vi "Steuerprogramm-12-15.vi"() -> ()   [LabVIEW 2010]
uses:
  <vilib>/rvi/interface/nirviReadWriteControl/nirviReadWriteControl.xnode
  <vilib>/rvi/errors/niLvFpgaWhatHappensToTopLevelVI.ctl
  <vilib>/rvi/interface/common/niFpgaNodeNameForErrorReporting.ctl
  <vilib>/rvi/errors/niLvFpgaAdjustHostInterfaceError.vi
  gvbooleschRT.vi
  <vilib>/rvi/interface/nirviCloseFPGA/nirviCloseFPGA.xnode
  GVMWHorst.vi
  GVMethodenwechsel.vi
  GVHorstSP.vi
  GVZwangs.vi
  GVHK1Hz.vi
  GVHeizenLH.vi
  GVAIs.vi
  GVTrapsMachs.vi
  GVaktuelleTDMS.vi
  GVECDs.vi
  GVZeitenZyklen.vi
  GVProbenvol.vi
  GVVentilposition.vi
  <vilib>/rvi/interface/nirviMethod/nirviMethod.xnode
  GVChroms.vi
  C:/Users/HAGAR-IV/Desktop/Zeugs/Johnny/pertrasgc fpga/FPGA-Programm-11-15.vi
  GVMetavariablen.vi
  GVZwangsMPV.vi
  C:/Users/HAGAR-IV/Desktop/Zeugs/markus/version feb 2012/FPGA Bitfiles/pertrasgcfpga2_FPGATarget_FPGA-Programm-11_875D3646.lvbitx
  NiFpgaLv.dll
  <vilib>/Utility/error.llb/Error Cluster From Error Code.vi
  <vilib>/FPGAPlugInAG/cRIO-9114/niLvFpga_Close_cRIO-9114.vi
  Emil/HAGAR V - Licor/control/Licor-Sequences.ctl
  Emil/HAGAR V - Licor/control/Licor-Pump.ctl
  Emil/Licor-Steuerung/LicorLI7000/conventions/Licor-Source.ctl
  Emil/Licor-Steuerung/LicorLI7000/LicorLI7000.lvlib
  Emil/HAGAR V - Licor/control/Licor-Parameter.ctl
panel:
  in  "Methode speichern":bool
  out "ZyklusNummernGesamt":i32[](array[numeric])
  in  "veränderte Methode benutzen":bool
  in  "Methode verändern":bool
  out "ZyklusNummern":i32[](array[numeric])
  out "Big Ben, Methodenzeit, Zykluszeit0, Zykluszeit1, Zykluszeit2A, Zykluszeit2B":i32[](array[numeric])
  in  "global stop RT":bool
  in  "Methode":i32(ring) items=["Bedingsmethode", "Startmethode", "Meßmodus", "Shut-up-Methode", "Test", "HAG2 1/2", "Startmethode", "HAG2 1/2 Aufwärmen"]
  in  "Registerkarte":T1(tab)
  out "AIs1":dbl[](array[numeric])
  out "AIs1":string[](array[string])
  out "AIs2":string[](array[string])
  out "AIs3":string[](array[string])
  out "AIs2":dbl[](array[numeric])
  out "AIs3":dbl[](array[numeric])
  out "Metavariablen":string[](array[string])
  out "Metavariablen":dbl[](array[numeric])
  out "MWHorst":dbl[](array[numeric])
  out "HorstRegler":string[](array[string])
  out "Ventilposition":i32=1 min=1 max=6 step=1
  out "Housekeeping1":cluster{dbl[], dbl[]}(graph)
  in  "Zeitachse1":i32(ring)=1 items=["Zykluszeit [s] Mod0", "Zykluszeit [s] Mod1", "Zykluszeit [s] Mod2A", "Zykluszeit [s] Mod2B"]
  in  "dargestellte Größe 1":i32(ring)=1 items=["T1-Trap1", "T1-Trap2", "T1-StirlingKühlkopf", "T1-PreCol1", "T1-PreCol2", "T1-MainCol1a", "T1-MainCol1b", "T1-MainCol2a", "T1-MainCol2b", "T1-Bronkhorst1a", "T1-Bronkhorst1b", "T1-Bronkhorst2a", "T1-Bronkhorst2b", "T1-2Pos1B", "T1-Spare9", "T1-2Pos1A", "T1-Spare10", "T1-TurboPump", "T1-StirlingPlatine", "T1-Spare5", "T1-Spare6", "T1-Spare7", "T1-Spare8", "F1-MFM1", "F1-MFM0D [mL]", "P1-MethaneHP", "P1-MethaneLP", "P1-Vacuum", "TurboSpeed", "I1-MS-AC", "I1-Trap1", "I1-Trap2", "T2-ECD1a", "T2-ECD1b", "T2-ECD2a", "T2-ECD2b", "T2-Col1a", "T2-Col1b", "T2-Col2a", "T2-Col2b", "T2-Spare1", "T2-Spare2", "T2-Oven_a", "T2-Oven_b", "T2-Spare3", "T2-Spare4", "T2-Spare5", "F2-MFM0", "F2-MFM2A", "F2-MFM2B", "P2-N2O_HP", "P2-N2O_LP", "P2-CO2_HP", "P2-CO2_LP", "AI-Spare1", "FL-MFM1000mL", "AI-Spare3", "AI-Spare4", "StirlingAlarm", "StirlingEmerg.", "AI-Spare7", "AI-Spare8", "AI-Spare9", "FL-MFM30mL", "T0-DC/DC5", "I0-24V_M0", "I0-48V_M1", "I0-24V_M1", "I0-28V_M2", "T0-Spare3", "T0-Spare2", "T0-Spare4", "T0-DC/DC7", "I0-20V_Laptop", "I0-28V_M1", "I0-24V_M2", "I0-12V_Licor", "T0-Spare1", "T0-Drier", "T0-Spare5", "F0-MFM0A [L]", "TL-Licor_a", "P0-Span-HP", "P0-spare1", "P0-Stickstoff-LP", "P0-Helium-LP", "P0-Cal-HP", "P0-P9Tavco[bar]", "F0-MFM0B [L]", "TL-Licor_b", "P0-Span-LP", "P0-spare2", "P0-Stickstoff-HP", "P0-Helium-HP", "P0-Cal-LP", "F0-MFM3", "TemperaturTrap1[°C]", "TemperaturTrap2[°C]", "TemperaturPreMach1[°C]", "TemperaturPreMach2[°C]", "TemperaturMainMach1[°C]", "TemperaturMainMach2[°C]", "PrC0", "PrC0-Licor", "PrC1-Säule2", "PrC1-Säule1", "MFC1-Sample", "MFC1-Methan", "PrC1-BackFlush1", "PrC1-BackFlush2", "MFC2A", "MFC2B", "MFC2C", "PrC2A", "MFC2D", "MFC2E", "PrC2B"]
  out "Housekeeping2":cluster{dbl[], dbl[]}(graph)
  in  "Zeitachse2":i32(ring)=1 items=["Zykluszeit [s] Mod0", "Zykluszeit [s] Mod1", "Zykluszeit [s] Mod2A", "Zykluszeit [s] Mod2B"]
  in  "dargestellte Größe 2":i32(ring)=1 items=["T1-Trap1", "T1-Trap2", "T1-StirlingKühlkopf", "T1-PreCol1", "T1-PreCol2", "T1-MainCol1a", "T1-MainCol1b", "T1-MainCol2a", "T1-MainCol2b", "T1-Bronkhorst1a", "T1-Bronkhorst1b", "T1-Bronkhorst2a", "T1-Bronkhorst2b", "T1-2Pos1B", "T1-Spare9", "T1-2Pos1A", "T1-Spare10", "T1-TurboPump", "T1-StirlingPlatine", "T1-Spare5", "T1-Spare6", "T1-Spare7", "T1-Spare8", "F1-MFM1", "F1-MFM0D [mL]", "P1-MethaneHP", "P1-MethaneLP", "P1-Vacuum", "TurboSpeed", "I1-MS-AC", "I1-Trap1", "I1-Trap2", "T2-ECD1a", "T2-ECD1b", "T2-ECD2a", "T2-ECD2b", "T2-Col1a", "T2-Col1b", "T2-Col2a", "T2-Col2b", "T2-Spare1", "T2-Spare2", "T2-Oven_a", "T2-Oven_b", "T2-Spare3", "T2-Spare4", "T2-Spare5", "F2-MFM0", "F2-MFM2A", "F2-MFM2B", "P2-N2O_HP", "P2-N2O_LP", "P2-CO2_HP", "P2-CO2_LP", "AI-Spare1", "FL-MFM1000mL", "AI-Spare3", "AI-Spare4", "StirlingAlarm", "StirlingEmerg.", "AI-Spare7", "AI-Spare8", "AI-Spare9", "FL-MFM30mL", "T0-DC/DC5", "I0-24V_M0", "I0-48V_M1", "I0-24V_M1", "I0-28V_M2", "T0-Spare3", "T0-Spare2", "T0-Spare4", "T0-DC/DC7", "I0-20V_Laptop", "I0-28V_M1", "I0-24V_M2", "I0-12V_Licor", "T0-Spare1", "T0-Drier", "T0-Spare5", "F0-MFM0A [L]", "TL-Licor_a", "P0-Span-HP", "P0-spare1", "P0-Stickstoff-LP", "P0-Helium-LP", "P0-Cal-HP", "P0-P9Tavco[bar]", "F0-MFM0B [L]", "TL-Licor_b", "P0-Span-LP", "P0-spare2", "P0-Stickstoff-HP", "P0-Helium-HP", "P0-Cal-LP", "F0-MFM3", "TemperaturTrap1[°C]", "TemperaturTrap2[°C]", "TemperaturPreMach1[°C]", "TemperaturPreMach2[°C]", "TemperaturMainMach1[°C]", "TemperaturMainMach2[°C]", "PrC0", "PrC0-Licor", "PrC1-Säule2", "PrC1-Säule1", "MFC1-Sample", "MFC1-Methan", "PrC1-BackFlush1", "PrC1-BackFlush2", "MFC2A", "MFC2B", "MFC2C", "PrC2A", "MFC2D", "MFC2E", "PrC2B"]
  out "Detektor 2":cluster{dbl[], dbl[]}[](graph)
  in  "Detektor":i32(ring) items=["ECD1", "ECD2"]
  in  "HK1YMin":dbl
  in  "HK1YMax":dbl=100.0
  in  "HK2YMin":dbl
  in  "HK2YMax":dbl=100.0
  in  "DetYMin":dbl
  in  "DetYMax":dbl=100.0
  out "schnelleAnzeige":cluster{dbl[], dbl[]}(graph)
  in  "TafelWischen!":bool
  in  "dargestellte Größe 3":i32(ring)=1 items=["TemperaturTrap1[°C]", "TemperaturTrap2[°C]", "TemperaturPreMach1[°C]", "TemperaturPreMach2[°C]", "TemperaturMainMach1[°C]", "TemperaturMainMach2[°C]", "PrC0", "PrC0-Licor", "PrC1-Säule2", "PrC1-Säule1", "MFC1-Sample", "MFC1-Methan", "PrC1-BackFlush1", "PrC1-BackFlush2", "MFC2A", "MFC2B", "MFC2C", "PrC2A", "MFC2D", "MFC2E", "PrC2B"]
  in  "An/Aus":bool
  in  "manual control":T3={"sequence manual"=enum."WAIT", "sequence manual ?"=FALSE}
  out "Licor-output":string[](array[string])
  out "graph":cluster{"X":dbl[], "Y":dbl[]}(graph)
  in  "Licor-parameter out":T4={"CO2 ref"=392.0, "CO2 span"=402.0, "H2O ref"=0.0, "H2O span"=0.0, "Zi"=1.2, "Zt"=0.0, "Zm"=0.0, "S"=1.0, "Temp [C]"=50.0, "Pressure [hPa]"=135.0, "Licor-Sources"=["CO2A W", "CO2B W", "H2OA W", "H2OB W", "T C", "T V", "P kPa", "P V", "RH %", "CO2A um/m", "CO2B um/m", "H2OA mm/m", "H2OB mm/m"], "Licor-Pump"="Off", "Zeitstempel"=timestamp(0 s since 1904-01-01)} {"Pressure [hPa]" format="%.2g"; "Temp [C]" format="%.2f"; "CO2 ref" format="%.2f"; "CO2 span" format="%.2g"; "H2O ref" format="%.2g"; "H2O span" format="%.2g"}
  in  "ServosWarmHigh (us)KaltHigh(us)":T7={"Servo1WarmHigh(us)"=1000, "Servo1KaltHigh(us)"=1000, "Servo2WarmHigh(us)"=2030, "Servo2KaltHigh(us)"=2030}
  out "KonfigLaden":errorcluster
  out "FPGAInit":errorcluster
  out "TDMSwriteECD1":errorcluster
  out "TDMSwriteECD2":errorcluster
  out "AIsFIFOread":errorcluster
  out "MWTrapsMachs":errorcluster
  out "TDMSwriteHK":errorcluster
  out "TDMSopenHK":errorcluster
  out "TDMScloseHK":errorcluster
  out "writeFIFORS485":errorcluster
  out "SeriellReadWrite":errorcluster
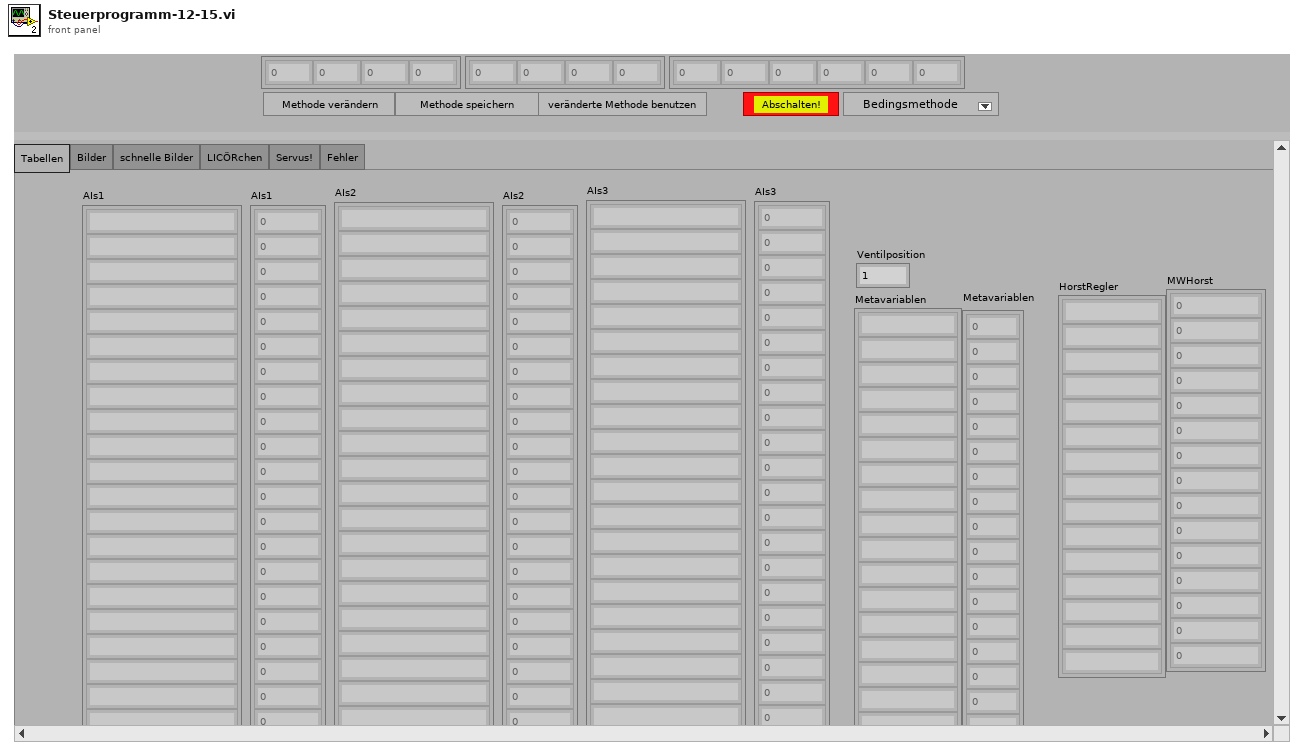
[diagram p1: front panel]
types:
  T1 = enum32{"Tabellen", "Bilder", "schnelle Bilder", "LICÖRchen", "Servus!", "Fehler"}
  T2 = typedef "Licor-Sequences.ctl" = enum16{"test", "WAIT", "warmup", "initialize", "calibrate Z", "calibrate S"}
  T3 = cluster{"sequence manual":T2, "sequence manual ?":bool}
  T4 = typedef "Licor-Parameter.ctl" = cluster{"CO2 ref":dbl, "CO2 span":dbl, "H2O ref":dbl, "H2O span":dbl, "Zi":dbl, "Zt":dbl, "Zm":dbl, "S":dbl, "Temp [C]":dbl, "Pressure [hPa]":dbl, "Licor-Sources":T5[], "Licor-Pump":T6, "Zeitstempel":timestamp}
  T5 = typedef "LicorLI7000.lvlib/Licor-Source.ctl" = string
  T6 = typedef "Licor-Pump.ctl" = string
  T7 = cluster{"Servo1WarmHigh(us)":u32, "Servo1KaltHigh(us)":u32, "Servo2WarmHigh(us)":u32, "Servo2KaltHigh(us)":u32}
  T8 = cluster{"DIOsMod0Nr":i32[], "DIOsMod1Nr":i32[], "DIOsMod2ANr":i32[], "DIOsMod2BNr":i32[], "AIsLH":i32[], "AnzahlRegler/Modul":i32[], "Regler für den Probenfluß":i32, "SPvorgebenMod0":string[], "SPvorgebenMod1":string[], "SPvorgebenMod2A":string[], "SPvorgebenMod2B":string[], "MWAntwortMod0":string[], "MWAntwortMod1":string[], "MWAntwortMod2A":string[], "MWAntwortMod2B":string[], "FaktorMod0":dbl[], "FaktorMod1":dbl[], "FaktorMod2A":dbl[], "FaktorMod2B":dbl[], "MWabfragenMod0":string[], "MWabfragenMod1":string[], "MWabfragenMod2A":string[], "MWabfragenMod2B":string[], "Modul1/AI koeff":dbl[][], "Modul2/AI koeff":dbl[][], "Modul3/AI koeff":dbl[][], "Traps/MachsKoeff":dbl[][], "Modul1/AIsNamen":string[], "Modul2/AIsNamen":string[], "Modul3/AIsNamen":string[], "DIOsMod0Name":string[], "DIOsMod1Name":string[], "DIOsMod2AName":string[], "DIOsMod2BName":string[], "ReglerNameMod0":string[], "ReglerNameMod1":string[], "ReglerNameMod2A":string[], "ReglerNameMod2B":string[], "Startmethode":i32, "Dateiordner Housekeeping":path, "Dateiname Housekeeping":string, "DateiordnerECD1":path, "DateinameECD1":string, "DateiordnerECD2":path, "DateinameECD2":string, "NamenLangsameHeizungen":string[], "ModuleLH":i32[], "Metavariablen":string[]}
  T9 = cluster{"Zykluslängen [s]":dbl[], "ZeitpktDIOsMod0":dbl[], "ZeitpktDIOsMod1":dbl[], "ZeitpktDIOsMod2A":dbl[], "ZeitpktDIOsMod2B":dbl[], "DIOsSPMod0":bool[][], "DIOsSPMod1":bool[][], "DIOsSPMod2A":bool[][], "DIOsSPMod2B":bool[][], "Mod0HorstZeitpkt":dbl[], "Mod1HorstZeitpkt":dbl[], "Mod2AHorstZeitpkt":dbl[], "Mod2BHorstZeitpkt":dbl[], "HorstSPMod0":dbl[][], "HorstSPMod1":dbl[][], "HorstSPMod2A":dbl[][], "HorstSPMod2B":dbl[][], "LHSetpoints":dbl[], "LHHeizen?":bool[], "ZPktFPGABoolesch":dbl[], "FPGABoolesch":bool[][], "ZeitpktFPGAPID":dbl[], "FPGAPID":cluster{"proportional gain (Kc)":fxp<+/-,16,8>, "integral gain (Kc*Ts/Ti)":fxp<+/-,16,8>, "derivative gain (Kc*Td/Ts)":fxp<+/-,16,8>}[][], "ZeitpktFPGAFixp":dbl[], "SHSetpoints":dbl[][], "t_PreMach1":dbl[], "T_PreMach1":dbl[], "t_PreMach2":dbl[], "T_PreMach2":dbl[], "PIDs für \"träge\" Heizungen":cluster{"proportional gain (Kc)":dbl, "integral time (Ti, min)":dbl, "derivative time (Td, min)":dbl}[], "Zwangsbedingungen":dbl[][], "Dateien fürs MS schicken?":bool, "ZeitpunkteMPV":dbl[], "SPMPV":i32[], "ZeitpktMS-1":dbl, "ZeitpktMS-2":dbl, "Int.Start1":dbl, "Int.Stop1":dbl, "Int.Start2":dbl, "Int.Stop2":dbl, "Methodenname":string, "t_MainMach1":dbl[], "T_MainMach1":dbl[], "t_MainMach2":dbl[], "T_MainMach2":dbl[]}[]
  T10 = enum16{"open", "replace", "create", "open or create", "replace or create", "replace or create with confirmation"}
  T11 = typedef "niFpgaNodeNameForErrorReporting.ctl" = enum16{"Open FPGA VI Reference", "Read/Write Control", "Invoke Method: Abort", "Invoke Method: Acknowledge IRQ", "Invoke Method: Download", "Invoke Method: FIFO.Configure", "Invoke Method: FIFO.Read", "Invoke Method: FIFO.Start", "Invoke Method: FIFO.Stop", "Invoke Method: FIFO.Write", "Invoke Method: Reset", "Invoke Method: Run", "Invoke Method: Wait on IRQ", "Close FPGA VI Reference"}
  T12 = typedef "niLvFpgaWhatHappensToTopLevelVI.ctl" = enum16{"top level VI scripted behind XNode", "top level VI inlined behind XNode"}
  T13 = cluster{"Zyklus1":i32, "Zeitachse1":i32, "dargestellte Größe 1":i32, "Zyklus2":i32, "Zeitachse2":i32, "dargestellte Größe 2":i32}
  T14 = cluster{"DIOsMod0Name":string[], "DIOsMod1Name":string[], "DIOsMod2AName":string[], "DIOsMod2BName":string[], "ReglerNameMod0":string[], "ReglerNameMod1":string[], "ReglerNameMod2A":string[], "ReglerNameMod2B":string[], "NamenLangsameHeizungen":string[]}
  T15 = cluster{"Zykluslängen [s]":dbl[], "ZeitpktDIOsMod0":dbl[], "ZeitpktDIOsMod1":dbl[], "ZeitpktDIOsMod2A":dbl[], "ZeitpktDIOsMod2B":dbl[], "DIOsSPMod0":bool[][], "DIOsSPMod1":bool[][], "DIOsSPMod2A":bool[][], "DIOsSPMod2B":bool[][], "Mod0HorstZeitpkt":dbl[], "Mod1HorstZeitpkt":dbl[], "Mod2AHorstZeitpkt":dbl[], "Mod2BHorstZeitpkt":dbl[], "HorstSPMod0":dbl[][], "HorstSPMod1":dbl[][], "HorstSPMod2A":dbl[][], "HorstSPMod2B":dbl[][], "LHSetpoints":dbl[], "LHHeizen?":bool[], "ZPktFPGABoolesch":dbl[], "FPGABoolesch":bool[][], "ZeitpktFPGAPID":dbl[], "FPGAPID":cluster{"proportional gain (Kc)":fxp<+/-,16,8>, "integral gain (Kc*Ts/Ti)":fxp<+/-,16,8>, "derivative gain (Kc*Td/Ts)":fxp<+/-,16,8>}[][], "ZeitpktFPGAFixp":dbl[], "SHSetpoints":dbl[][], "t_PreMach1":dbl[], "T_PreMach1":dbl[], "t_PreMach2":dbl[], "T_PreMach2":dbl[], "PIDs für \"träge\" Heizungen":cluster{"proportional gain (Kc)":dbl, "integral time (Ti, min)":dbl, "derivative time (Td, min)":dbl}[], "Zwangsbedingungen":dbl[][], "Dateien fürs MS schicken?":bool, "ZeitpunkteMPV":dbl[], "SPMPV":i32[], "ZeitpktMS-1":dbl, "ZeitpktMS-2":dbl, "Int.Start1":dbl, "Int.Stop1":dbl, "Int.Start2":dbl, "Int.Stop2":dbl, "Methodenname":string, "t_MainMach1":dbl[], "T_MainMach1":dbl[], "t_MainMach2":dbl[], "T_MainMach2":dbl[]}
  T16 = cluster{"created path":path, "created path":path, "created path":path, "Dateiname Housekeeping":string, "DateinameECD1":string, "DateinameECD2":string, "tdms0":refnum<k34>, "tdms1":refnum<k34>, "tdms0":refnum<k34>, "tdms1":refnum<k34>, "tdms0":refnum<k34>, "tdms1":refnum<k34>}
  T17 = cluster{"proportional gain (Kc)":fxp<+/-,16,8>, "integral gain (Kc*Ts/Ti)":fxp<+/-,16,8>, "derivative gain (Kc*Td/Ts)":fxp<+/-,16,8>}[][]
  T18 = cluster{"proportional gain (Kc)":dbl, "integral time (Ti, min)":dbl, "derivative time (Td, min)":dbl}[]
  T19 = cluster{cluster{"ZeitpktDIOsMod2B":dbl[]}[], cluster{"DIOsSPMod2B":bool[][]}[], cluster{"Mod2BHorstZeitpkt":dbl[]}[], cluster{"HorstSPMod2B":dbl[][]}[], "LHHeizen?":bool[], "ZPktFPGABoolesch":dbl[], "FPGABoolesch":bool[][], "ZeitpktFPGAPID":dbl[], "FPGAPID":cluster{"proportional gain (Kc)":fxp<+/-,16,8>, "integral gain (Kc*Ts/Ti)":fxp<+/-,16,8>, "derivative gain (Kc*Td/Ts)":fxp<+/-,16,8>}[][], "ZeitpktFPGAFixp":dbl[], "SHSetpoints":dbl[][], "t_PreMach1":dbl[], "T_PreMach1":dbl[], "t_PreMach2":dbl[], "T_PreMach2":dbl[], "ZeitpunkteMPV":dbl[], "SPMPV":i32[], "t_MainMach1":dbl[], "T_MainMach1":dbl[], "t_MainMach2":dbl[], "T_MainMach2":dbl[]}
  T20 = cluster{"Zykluslängen [s]":dbl[], "ZeitpktDIOsMod0":dbl[], "ZeitpktDIOsMod1":dbl[], "ZeitpktDIOsMod2A":dbl[], "ZeitpktDIOsMod2B":dbl[], "DIOsSPMod0":bool[][], "DIOsSPMod1":bool[][], "DIOsSPMod2A":bool[][], "DIOsSPMod2B":bool[][], "Mod0HorstZeitpkt":dbl[], "Mod1HorstZeitpkt":dbl[], "Mod2AHorstZeitpkt":dbl[], "Mod2BHorstZeitpkt":dbl[], "HorstSPMod0":dbl[][], "HorstSPMod1":dbl[][], "HorstSPMod2A":dbl[][], "HorstSPMod2B":dbl[][], "LangsameHeizungenSP":dbl[], "LHHeizen?":bool[], "ZPktFPGABoolesch":dbl[], "FPGABoolesch":bool[][], "ZeitpktFPGAPID":dbl[], "FPGAPID":cluster{"proportional gain (Kc)":fxp<+/-,16,8>, "integral gain (Kc*Ts/Ti)":fxp<+/-,16,8>, "derivative gain (Kc*Td/Ts)":fxp<+/-,16,8>}[][], "ZeitpktFPGAFixp":dbl[], "FPGAFixp":dbl[][], "t_PreMach1":dbl[], "T_PreMach1":dbl[], "t_PreMach2":dbl[], "T_PreMach2":dbl[], "PIDs für \"träge\" Heizungen":cluster{"proportional gain (Kc)":dbl, "integral time (Ti, min)":dbl, "derivative time (Td, min)":dbl}[], "Zwangsbedingungen":dbl[][], "MS-Daten?":bool, "ZeitpunkteMPV":dbl[], "SetpointMPV":i32[], "ZeitpktMS-1":dbl, "ZeitpktMS-2":dbl, "Int.Start1":dbl, "Int.Stop1":dbl, "Int.Start2":dbl, "Int.Stop2":dbl, "Methodenname":string, "t_MainMach1":dbl[], "T_MainMach1":dbl[], "t_MainMach2":dbl[], "T_MainMach2":dbl[]}
  T21 = cluster{"ZyklusNummern":i32[], "ZeilennummernDIOs":i32[], "ZwangsDIO?":cluster{bool[]}[], "ZeilennummernHorst":i32[], "ZwangsHorst?":cluster{bool[]}[], "ZeileFPGABoolesch":i32, "ZwangsFPGABoolesch?":bool[], "ZeileFPGAPID":i32, "ZeileFPGAFixp":i32, "ZeilePreMach1":i32, "ZeilePreMach2":i32, "ZeilennummerMPV":i32, "ZeileMainMach1":i32, "ZeileMainMach2":i32, "ZwangsMPV?":bool}
  T22 = cluster{"ZyklusNummern":i32[], i32[], "ZwangsDIO?":cluster{bool[]}[], i32[], "ZwangsHorst?":cluster{bool[]}[], i32, "ZwangsFPGABoolesch?":bool[], i32, i32, "ZeileMach":i32, "ZeileMach":i32, i32, "ZeileMach":i32, "ZeileMach":i32, "ZwangsMPV?":bool}
  T23 = cluster{string[], string[], string[], dbl[], dbl[], dbl[]}
  T24 = cluster{"Befehle1":string[], "Befehle2":string[], "Befehle3":string[]}
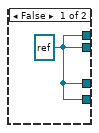
[diagram p2: hidden frame]
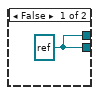
[diagram p3: hidden frame]
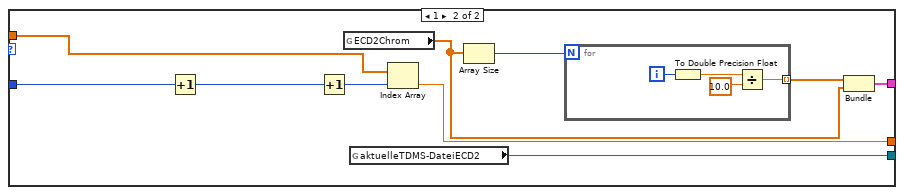
[diagram p13: hidden frame]
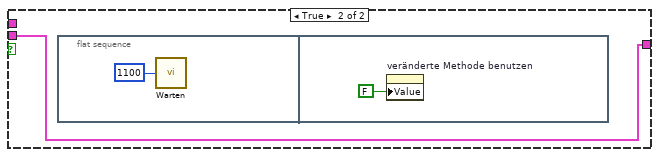
[diagram p14: hidden frame]
diagram:
  n1 = Open/Create/Replace File(file path (use dialog)=path "c:/einstellungen.per" ("Datei (Dialog verwenden)"), error in=errorcluster {"status"=FALSE, "code"=0, "source"=""}, operation (0:open)=T10."open" ("Operation (0:Öffnen)")) -> (refnum out=w19:refnum<file>, error out=w7:errorcluster)  [unwired: 3 in, 1 out]
  n2 = Read from Binary File(5:T8 {"DIOsMod0Nr"=[], "DIOsMod1Nr"=[], "DIOsMod2ANr"=[], "DIOsMod2BNr"=[], "AIsLH"=[], "AnzahlRegler/Modul"=[], "Regler für den Probenfluß"=0, "SPvorgebenMod0"=[], "SPvorgebenMod1"=[], "SPvorgebenMod2A"=[], "SPvorgebenMod2B"=[], "MWAntwortMod0"=[], "MWAntwortMod1"=[], "MWAntwortMod2A"=[], "MWAntwortMod2B"=[], "FaktorMod0"=[], "FaktorMod1"=[], "FaktorMod2A"=[], "FaktorMod2B"=[], "MWabfragenMod0"=[], "MWabfragenMod1"=[], "MWabfragenMod2A"=[], "MWabfragenMod2B"=[], "Modul1/AI koeff"=[], "Modul2/AI koeff"=[], "Modul3/AI koeff"=[], "Traps/MachsKoeff"=[], "Modul1/AIsNamen"=[], "Modul2/AIsNamen"=[], "Modul3/AIsNamen"=[], "DIOsMod0Name"=[], "DIOsMod1Name"=[], "DIOsMod2AName"=[], "DIOsMod2BName"=[], "ReglerNameMod0"=[], "ReglerNameMod1"=[], "ReglerNameMod2A"=[], "ReglerNameMod2B"=[], "Startmethode"=0, "Dateiordner Housekeeping"=path "", "Dateiname Housekeeping"="", "DateiordnerECD1"=path "", "DateinameECD1"="", "DateiordnerECD2"=path "", "DateinameECD2"="", "NamenLangsameHeizungen"=[], "ModuleLH"=[], "Metavariablen"=[]} ("Ausgangs-Cluster"), 8:w7, 11:w19) -> (0:w6:errorcluster, 2:w17:T8, 3:w18:refnum<file>)  [unwired: 3 in, 1 out]
  n3 = Close File(refnum=w18, error in=w6) -> (error out=w5:errorcluster)  [unwired: 1 out]
  n4 = Open/Create/Replace File(file path (use dialog)=path "c:/methoden.per" ("Datei (Dialog verwenden)"), error in=w5, operation (0:open)=T10."open" ("Operation (0:Öffnen)")) -> (refnum out=w14:refnum<file>, error out=w4:errorcluster)  [unwired: 3 in, 1 out]
  n5 = Read from Binary File(5:T9 [], 8:w4, 11:w14) -> (0:w3:errorcluster, 2:w12:T9, 3:w13:refnum<file>)  [unwired: 3 in, 1 out]
  n6 = Close File(refnum=w13, error in=w3) -> (error out=→"KonfigLaden":errorcluster)  [unwired: 1 out]
  n7 = flat-sequence {
    tunnel: [w102] -> w46
    tunnel: [w107] -> w45
    tunnel: [w241] -> w43
    tunnel: [w243] -> w42
    tunnel: [w235] -> w41
    tunnel: [w242] -> w40
    tunnel: [w165] -> w39
    tunnel: [w234] -> w38
    tunnel: [w233] -> w37
    tunnel: [w227] -> w36
    tunnel: [w168] -> w35
    tunnel: [w142] -> w34
    tunnel: [w240] -> w33
    tunnel: [w232] -> w32
    tunnel: [w231] -> w31
    tunnel: [w223] -> w30
    tunnel: [w222] -> w29
    tunnel: [w221] -> w28
    tunnel: [w220] -> w27
    tunnel: [w219] -> w26
    tunnel: [w218] -> w25
    tunnel: [w215] -> w24
    tunnel: [w197] -> w23
    tunnel: w17 -> [w81]
    tunnel: [w196] -> w22
    tunnel: w12 -> [w108]
    tunnel: [w107] -> w11
    tunnel: [w81] -> w8
    tunnel: w46 -> [w439]
    tunnel: w45 -> [w512]
    tunnel: [w439] -> w44
    tunnel: w43 -> [w470]
    tunnel: w42 -> [w469]
    tunnel: w41 -> [w471]
    tunnel: w40 -> [w468]
    tunnel: w39 -> [w443]
    tunnel: w38 -> [w438]
    tunnel: w37 -> [w435]
    tunnel: w36 -> [w432]
    tunnel: w35 -> [w433]
    tunnel: w34 -> [w436]
    tunnel: w33 -> [w510]
    tunnel: w32 -> [w441]
    tunnel: w31 -> [w511]
    tunnel: w30 -> [w414]
    tunnel: w29 -> [w413]
    tunnel: w28 -> [w412]
    tunnel: w27 -> [w508]
    tunnel: w26 -> [w507]
    tunnel: w25 -> [w506]
    tunnel: w24 -> [w460]
    tunnel: w23 -> [w442]
    tunnel: w22 -> [w431]
    tunnel: w12 -> [w430]
    tunnel: w11 -> [w428]
    tunnel: w8 -> [_]
    tunnel: w44 -> [w1264]
    frame #0 {
      w109 = TRUE
      w124 = 0.0 ("Probenvol.1")
      w131 = dbl[] [-1.0] ("ECD1MW")
      w132 = FALSE ("ECD1Empfangen?")
      w123 = string[] ["TemperaturTrap1[°C]", "TemperaturTrap2[°C]", "TemperaturPreMach1[°C]", "TemperaturPreMach2[°C]", "TemperaturMainMach1[°C]", "TemperaturMainMach2[°C]"]
      w238 = string[] ["Big Ben [s]", "Methodenzeit [s]", "Zykluszeit [s] Mod0", "Zykluszeit [s] Mod1", "Zykluszeit [s] Mod2A", "Zykluszeit [s] Mod2B"]
      w228 = FALSE ("Undefinierte Werte möglich")
      w229 = FALSE ("global stop RT")
      n8 = for {
        tunnel: [w403] -> w236 mode=indexing
        tunnel: w108 -> [w404] mode=indexing
        n9 = Unbundle(w404) -> ("Methodenname"=w403:string)  [unwired: 44 out]
      }
      n10 = Unbundle(w81) -> ("DIOsMod0Nr"=w152:i32[], "DIOsMod1Nr"=w151:i32[], "DIOsMod2ANr"=w150:i32[], "DIOsMod2BNr"=w149:i32[], "AIsLH"=w139:i32[], "AnzahlRegler/Modul"=w142:i32[], "Regler für den Probenfluß"=w196:i32, "SPvorgebenMod0"=w195:string[], "SPvorgebenMod1"=w194:string[], "SPvorgebenMod2A"=w193:string[], "SPvorgebenMod2B"=w192:string[], "MWAntwortMod0"=w191:string[], "MWAntwortMod1"=w190:string[], "MWAntwortMod2A"=w189:string[], "MWAntwortMod2B"=w188:string[], "FaktorMod0"=w187:dbl[], "FaktorMod1"=w186:dbl[], "FaktorMod2A"=w185:dbl[], "FaktorMod2B"=w184:dbl[], "MWabfragenMod0"=w183:string[], "MWabfragenMod1"=w182:string[], "MWabfragenMod2A"=w181:string[], "MWabfragenMod2B"=w180:string[], "Modul1/AI koeff"=w179:dbl[][], "Modul2/AI koeff"=w178:dbl[][], "Modul3/AI koeff"=w177:dbl[][], "Traps/MachsKoeff"=w176:dbl[][], "Modul1/AIsNamen"=w175:string[], "Modul2/AIsNamen"=w174:string[], "Modul3/AIsNamen"=w173:string[], "DIOsMod0Name"=w79:string[], "DIOsMod1Name"=w80:string[], "DIOsMod2AName"=w78:string[], "DIOsMod2BName"=w77:string[], "ReglerNameMod0"=w96:string[], "ReglerNameMod1"=w95:string[], "ReglerNameMod2A"=w94:string[], "ReglerNameMod2B"=w93:string[], "Startmethode"=w107:i32, "Dateiordner Housekeeping"=w76:path, "Dateiname Housekeeping"=w172:string, "DateiordnerECD1"=w90:path, "DateinameECD1"=w171:string, "DateiordnerECD2"=w89:path, "DateinameECD2"=w170:string, "NamenLangsameHeizungen"=w169:string[], "ModuleLH"=w164:i32[], "Metavariablen"=w100:string[])
      "Metavariablen" <- w100
      n11 = call "FPGA-Start-11-15.vi"() -> ("error out"=w50:errorcluster, "FPGA VI Reference Out"=w58:refnum<k20>)  [unwired: 2 in]
      n12 = Initialize Array(0, 4 ("Dimension")) -> (w125:i32[])
      n13 = Initialize Array(0.0 ("Element"), 6 ("Dimension")) -> (w128:dbl[])
      n14 = global write "GVMethodenwechsel.vi" "Methodenwechsel?"(FALSE ("Methodenwechsel?")) -> ()
      n15 = Concatenate Strings("?SE0,SETP,2200" ("string"), "\r\n") -> (w52:string)
      n16 = Concatenate Strings("?SE0,SETP,2300" ("string"), "\r\n") -> (w60:string)
      n17 = String To Byte Array(string=w60) -> (unsigned byte array=w66:u8[])
      n18 = Join Numbers(hi=w66, lo=u8 6) -> ((hi.lo)=w64:u16[])
      n19 = String To Byte Array(string=w52) -> (unsigned byte array=w54:u8[])
      n20 = Join Numbers(hi=w54, lo=u8 5) -> ((hi.lo)=w51:u16[])
      n21 = xnode "Invoke Method"("FPGA VI Reference In"=w58, "error in"=w50, "Data"=w51) -> ("FPGA VI Reference Out"=w57:refnum<k20>, "error out"=w49:errorcluster)  [unwired: 1 in, 1 out]
      n22 = xnode "Invoke Method"("FPGA VI Reference In"=w57, "error in"=w49, "Data"=w64) -> ("FPGA VI Reference Out"=w63:refnum<k20>, "error out"=w48:errorcluster)  [unwired: 1 in, 1 out]
      n23 = global write "GVProbenvol.vi" "Probenvol.1"(w124) -> ()
      n24 = global write "GVProbenvol.vi" "Probenvol.2"(w124) -> ()
      n25 = global write "GVECDs.vi" "ECD1MW"(w131) -> ()
      n26 = global write "GVECDs.vi" "ECD2MW"(w131) -> ()
      n27 = global write "GVECDs.vi" "ECD1Empfangen?"(w132) -> ()
      n28 = global write "GVECDs.vi" "ECD2Empfangen?"(w132) -> ()
      n29 = property on="dargestellte Größe 2" class="Ring (strict)"("AllowUndefVals"=w228) -> ()  [unwired: 2 in, 2 out]
      n30 = property on="Zeitachse2" class="Ring (strict)"("AllowUndefVals"=w228) -> ()  [unwired: 2 in, 2 out]
      n31 = property on="Zeitachse1" class="Ring (strict)"("AllowUndefVals"=w228) -> ()  [unwired: 2 in, 2 out]
      n32 = property on="dargestellte Größe 1" class="Ring (strict)"("AllowUndefVals"=w228) -> ()  [unwired: 2 in, 2 out]
      n33 = property on="Methode" class="Ring (strict)"("AllowUndefVals"=w228) -> ()  [unwired: 2 in, 2 out]
      n34 = local write "global stop RT"(w229) -> ()
      n35 = global write "gvbooleschRT.vi" "global stop RT"(w229) -> ()
      n36 = global write "GVZeitenZyklen.vi" "ZyklusNummern"(w125) -> ()
      n37 = global write "GVZeitenZyklen.vi" "ZyklusNummernGesamt"(w125) -> ()
      n38 = global write "GVZeitenZyklen.vi" "Big Ben, Methodenzeit, Zykluszeit0, Zykluszeit1, Zykluszeit2A, Zykluszeit2B"(w128) -> ()
      n39 = property on="Methode" class="Ring (strict)"("Value"=w107) -> ()  [unwired: 2 in, 2 out]
      n40 = Initialize Array(-1.0 ("Element"), 6 ("Dimension")) -> (w135:dbl[])
      n41 = Initialize Array(FALSE, 10 ("Dimension")) -> (w143:bool[])
      n42 = Initialize Array(-1.0 ("Element"), 96 ("Dimension")) -> (w136:dbl[])
      n43 = call "MPVSenden-11-15.vi"("Ventilposition"=0, "error in"=w48, "FPGA VI Reference In"=w63) -> ("error out"=→"FPGAInit":errorcluster, "FPGA VI Reference Out"=w102:refnum<k20>)  [unwired: 1 out]
      n44 = global write "GVZwangs.vi" "ZwangsFPGABoolesch!"(w143) -> ()
      n45 = global write "GVZwangs.vi" "ZwangsFPGABoolesch?"(w143) -> ()
      n46 = global write "GVTrapsMachs.vi" "Traps/Machs"(w135) -> ()
      n47 = global write "GVAIs.vi" "AIs"(w136) -> ()
      n48 = for {
        tunnel: w142 -> [w381] mode=indexing
        tunnel: [w378] -> w141 mode=indexing
        tunnel: [w376] -> w140 mode=indexing
        n49 = Initialize Array(0.0 ("Element"), w381) -> (w379:dbl[])
        n50 = Initialize Array(FALSE, w381) -> (w377:bool[])
        n51 = Bundle(w379) -> (w378:cluster{dbl[]})  [unwired: 1 in]
        n52 = Bundle(w377) -> (w376:cluster{bool[]})  [unwired: 1 in]
      }
      n53 = Bundle("DIOsMod0Name"=w79, "DIOsMod1Name"=w80, "DIOsMod2AName"=w78, "DIOsMod2BName"=w77, "ReglerNameMod0"=w96, "ReglerNameMod1"=w95, "ReglerNameMod2A"=w94, "ReglerNameMod2B"=w93, "NamenLangsameHeizungen"=w169) -> (w231:T14)  [unwired: 1 in]
      n54 = Build Array (concatenate)(w96, w95, w94, w93) -> (w122:string[])
      n55 = Build Array (concatenate)(w191, w190, w189, w188) -> (w242:string[])
      n56 = Build Array (concatenate)(w195, w194, w193, w192) -> (w243:string[])
      n57 = Build Array (concatenate)(w187, w186, w185, w184) -> (w235:dbl[])
      n58 = Build Array (concatenate)(w183, w182, w181, w180) -> (w241:string[])
      n59 = Build Array (concatenate)(w96, w95, w94, w93) -> (→"HorstRegler":string[])
      n60 = Array Size(array=w100) -> (size(s)=w99:i32)
      n61 = Build Array(w152, w151, w150, w149) -> (w148:i32[][])
      n62 = Array Size(array=w169) -> (size(s)=w168:i32)
      n63 = Add Array Elements(numeric array=w142) -> (sum=w227:i32)
      n64 = Array Size(array=w139) -> (size(s)=w138:i32)
      n65 = Index Array(array=w108, index=w107) -> (element=w106:T15)
      n66 = Add Array Elements(numeric array=w142) -> (sum=w154:i32)
      n67 = Build Cluster Array(w152, w151, w150, w149) -> (w234:cluster{"DIOsMod2BNr":i32[]}[])
      n68 = Decrement(x=w164) -> (x-1=w163:i32[])
      n69 = Build Array (concatenate)(w175, w174, w173) -> (w113:string[])
      n70 = Index Array(array=w176, index (col)=0 ("Deaktivierter Index (Spalte)")) -> (element=w221:dbl[])  [unwired: 1 in]
      n71 = Index Array(array=w176, index (col)=1 ("Deaktivierter Index (Spalte)")) -> (element=w222:dbl[])  [unwired: 1 in]
      n72 = Index Array(array=w176, index (col)=2 ("Deaktivierter Index (Spalte)")) -> (element=w223:dbl[])  [unwired: 1 in]
      n73 = for {
        tunnel: w234 -> [w406] mode=indexing
        tunnel: [w407] -> w233 mode=indexing
        n74 = Unbundle(w406) -> ("DIOsMod2BNr"=w405:i32[])
        n75 = Array Size(array=w405) -> (size(s)=w407:i32)
      }
      n76 = property on="Methode" class="Ring (strict)"("Strings []"=w236) -> ()  [unwired: 2 in, 2 out]
      n77 = Build Array (concatenate)(w136, w135) -> (w134:dbl[])
      n78 = Array Size(array=w148) -> (size(s)=w147:i32[])
      n79 = Unbundle(w106) -> ("SPMPV"=w105:i32[])  [unwired: 44 out]
      n80 = Open/Create/Replace File(file path (use dialog)=path "c:/fromcriordy.txt" ("Dateipfad (Dialog verwenden)"), operation (0:open)=T10."replace or create" ("Operation (0:Öffnen)")) -> (refnum out=w200:refnum<file>, error out=w201:errorcluster)  [unwired: 4 in, 1 out]
      n81 = Initialize Array(0.0 ("Element"), w154) -> (w153:dbl[])
      n82 = Initialize Array(0.0 ("element"), w99) -> (w97:dbl[])
      n83 = Get Date/Time In Seconds() -> (seconds since 1Jan1904=w91:timestamp)
      n84 = Initialize Array(FALSE, w138) -> (w133:bool[])
      n85 = Multiply(x=w163, y=32) -> (x*y=w166:i32[])
      n86 = Initialize Array(-1.0, w154) -> (w156:dbl[])
      n87 = Array Subset(array=w113, index=32 ("Index"), length=32 ("Länge")) -> (→"AIs2":string[])
      n88 = Array Subset(array=w113, index=0 ("Index"), length=32 ("Länge")) -> (→"AIs1":string[])
      n89 = Array Subset(array=w113, index=64 ("Index"), length=32 ("Länge")) -> (→"AIs3":string[])
      n90 = global write "GVHK1Hz.vi" "Mod1Mod2Mod3/AITrapsMachs1Hz"(w134) -> ()
      n91 = global write "GVHorstSP.vi" "HorstSP"(w153) -> ()
      n92 = for {
        tunnel: w147 -> [w386] mode=indexing
        tunnel: [w383] -> w146 mode=indexing
        n93 = Initialize Array(FALSE, w386) -> (w384:bool[])
        n94 = Bundle(w384) -> (w383:cluster{bool[]})  [unwired: 1 in]
      }
      n95 = global write "GVMetavariablen.vi" "Metavariablen"(w97) -> ()
      n96 = global write "GVHeizenLH.vi" "Heizen?LH"(w133) -> ()
      n97 = global write "GVZwangs.vi" "ZwangsLangsameH!"(w133) -> ()
      n98 = global write "GVZwangs.vi" "ZwangsLangsameH?"(w133) -> ()
      n99 = Add(x=w166, y=w139) -> (x+y=w165:i32[])
      n100 = Close File(refnum=w200, error in=w201) -> (path=w232:path)  [unwired: 1 out]
      n101 = Format Date/Time String(time format string (%c)="%Y-%m-%d--%H-%M" ("Zeitformatierungs-String (%c)"), seconds (now)=w91) -> (date/time string=w69:string)  [unwired: 1 in]
      n102 = Index Array(array=w105, index=0) -> (element=w103:i32)
      n103 = global write "GVMWHorst.vi" "MWHorst"(w156) -> ()
      n104 = global write "GVVentilposition.vi" "Ventilposition"(w103) -> ()
      n105 = Build Array (concatenate)(string[] ["Jahr", "Monat", "Tag", "Stunde", "Minute", "Sekunde"] ("Array"), string[] ["Datei Nr.", "Methode Nr.", "Zyklusnr. Mod0", "Zyklusnr. Mod1", "Zyklusnr. Mod2A", "Zyklusnr. Mod2B"], w238, w113, w123, w122, "Probenvolumen1", "Probenvolumen2", "Ventilposition" ("element"), string[] ["CPU Total", "CPU Time critical", "CPU Timed Structures", "CPU High", "CPU Above normal", "CPU Normal", "CPU Background", "CPU Idle", "CPU ISR", "Memory", "SekundenTotalBrutal"]) -> (w240:string[])
      n106 = Build Array (concatenate)(w123, w122) -> (w121:string[])
      n107 = Build Array (concatenate)(w113, w123, w122) -> (w120:string[])
      n108 = Split 1D Array(array=w238, index=2 ("Index")) -> (second subarray=w230:string[])  [unwired: 1 out]
      n109 = Concatenate Strings("HK " ("String"), w69) -> (w73:string)
      n110 = Concatenate Strings("ECD1 " ("String"), w69) -> (w71:string)
      n111 = Concatenate Strings("ECD2 " ("String"), w69) -> (w68:string)
      n112 = property on="dargestellte Größe 1" class="Ring (strict)"("Strings []"=w120) -> ()  [unwired: 2 in, 2 out]
      n113 = property on="Zeitachse2" class="Ring (strict)"("Strings []"=w230) -> ()  [unwired: 2 in, 2 out]
      n114 = property on="Zeitachse1" class="Ring (strict)"("Strings []"=w230) -> ()  [unwired: 2 in, 2 out]
      n115 = property on="dargestellte Größe 3" class="Ring (strict)"("Strings []"=w121) -> ()  [unwired: 2 in, 2 out]
      n116 = global write "GVZwangs.vi" "ZwangsHorst!"(w141) -> ()
      n117 = property on="dargestellte Größe 2" class="Ring (strict)"("Strings []"=w120) -> ()  [unwired: 2 in, 2 out]
      n118 = global write "GVZwangs.vi" "ZwangsHorst?"(w140) -> ()
      n119 = Build Path(base path=w76, name or relative path=w73) -> (appended path=w84:path)
      n120 = Build Path(base path=w90, name or relative path=w71) -> (appended path=w86:path)
      n121 = Build Path(base path=w89, name or relative path=w68) -> (appended path=w88:path)
      n122 = Create Folder(path (use dialog)=w84) -> (created path=w83:path)  [unwired: 2 in, 2 out]
      n123 = Create Folder(path (use dialog)=w86) -> (created path=w85:path)  [unwired: 2 in, 2 out]
      n124 = Create Folder(path (use dialog)=w88) -> (created path=w87:path)  [unwired: 2 in, 2 out]
      n125 = global write "GVZwangs.vi" "ZwangsDIO!"(w146) -> ()
      n126 = global write "GVZwangs.vi" "ZwangsDIO?"(w146) -> ()
      n127 = case shown="True" w109 {
        tunnel: [w397 w402] -> w214
        tunnel: [w397 w401] -> w213
        tunnel: w83 -> [_ w400]
        tunnel: w172 -> [_ w399]
        tunnel: w107 -> [_ w398]
        frame False {
          w397 = refnum<k34> refnum ("tdms1")
        }
        frame True {
          n128 = call "TDMS0.vi"("Startmethode"=w398, "Dateiname"=w399, "Dateiordner"=w400) -> ("tdms1"=w401:refnum<k34>, "tdms0"=w402:refnum<k34>)
          n129 = global write "GVaktuelleTDMS.vi" "aktuelleTDMS-DateiHK"(w402) -> ()
        }
      }
      n130 = case shown="True" w109 {
        tunnel: [w387 w396] -> w212
        tunnel: [w387 w395] -> w211
        tunnel: [w387 w394] -> w210
        tunnel: [w387 w393] -> w209
        tunnel: w85 -> [_ w392]
        tunnel: w171 -> [_ w391]
        tunnel: w87 -> [_ w390]
        tunnel: w170 -> [_ w389]
        tunnel: w107 -> [_ w388]
        frame False {
          w387 = refnum<k34> refnum ("tdms0")
        }
        frame True {
          n131 = call "TDMS0.vi"("Startmethode"=w388, "Dateiname"=w391, "Dateiordner"=w392) -> ("tdms1"=w395:refnum<k34>, "tdms0"=w396:refnum<k34>)
          n132 = call "TDMS0.vi"("Startmethode"=w388, "Dateiname"=w389, "Dateiordner"=w390) -> ("tdms1"=w393:refnum<k34>, "tdms0"=w394:refnum<k34>)
          n133 = global write "GVaktuelleTDMS.vi" "aktuelleTDMS-DateiECD1"(w396) -> ()
          n134 = global write "GVaktuelleTDMS.vi" "aktuelleTDMS-DateiECD2"(w394) -> ()
        }
      }
      n135 = Open/Create/Replace File(file path (use dialog)=path "c:/fromcriocmd.txt" ("Pfad MS-Datei CRIO"), operation (0:open)=T10."replace or create" ("Operation (0:Öffnen)")) -> (refnum out=w206:refnum<file>, error out=w205:errorcluster)  [unwired: 4 in, 1 out]
      n136 = call "AIKoeffSortieren.vi"("Modul3/AI koeff"=w177, "Modul2/AI koeff"=w178, "Modul1/AI koeff"=w179) -> ("P0"=w218:dbl[], "P1"=w219:dbl[], "P2"=w220:dbl[])
      n137 = Write to Text File(file (use dialog)=w206, text="time=yyyymmddhhmmss\ncycle=005\ninfo=1234567890123456789012345678901234567890123456789012345678901234567890123456789012345678901234567890\nlength=100\ncmd=cycle" ("Text0 MS-Datei"), error in=w205) -> (refnum out=w203:refnum<file>, error out=w202:errorcluster)  [unwired: 1 in, 1 out]
      n138 = Bundle("created path"=w83, "created path"=w85, "created path"=w87, "Dateiname Housekeeping"=w172, "DateinameECD1"=w171, "DateinameECD2"=w170, "tdms0"=w214, "tdms1"=w213, "tdms0"=w212, "tdms1"=w211, "tdms0"=w210, "tdms1"=w209) -> (w215:T16)  [unwired: 1 in]
      n139 = Close File(refnum=w203, error in=w202) -> (path=w197:path)  [unwired: 1 out]
    }
    frame #1 {
      w415 = dbl[] [-1.0]
      w486 = 0
      w461 = 0 ("Zyklusnummer1")
      n140 = flat-sequence {
        frame #0 {
          n141 = control-ref of="graph"() -> (w513:refnum<vi>)
          n142 = control-ref of="manual control"() -> (w517:refnum<vi>)
          n143 = control-ref of="Licor-output"() -> (w516:refnum<vi>)
          n144 = control-ref of="Licor-parameter out"() -> (w515:refnum<vi>)
          n145 = call "licore (main).vi"(5:"Licor-parameter"=w515, "manual control"=w517, "raw data"=w516, 10:"Licor-parameter"="Licor-parameter out", "graph"=w513) -> ()  [unwired: 7 in]
        }
      }
      n146 = while {
        stop <- w1245 stop-if-true
        w1239 = 10.0
        n147 = call "Warten2"("Count(mSec)"=u32 1000) -> ()  [unwired: 1 out]
        n148 = global read "gvbooleschRT.vi" "global stop RT"() -> (w1245:bool)
        n149 = global read "GVTrapsMachs.vi" "Traps/Machs"() -> (w1235:dbl[])
        n150 = global read "GVAIs.vi" "AIs"() -> (w1236:dbl[])
        n151 = for {
          N: 9 -> [_]
          shift-right: [w1248] -> w1242
          shift-left: w1236 -> [w1249]
          shift-right: [w1246] -> w1240
          shift-left: w1235 -> [w1247]
          n152 = flat-sequence {
            tunnel: w1249 -> [w1256]
            tunnel: [w1255] -> w1248
            tunnel: w1247 -> [w1254]
            tunnel: [w1253] -> w1246
            frame #0 {
              n153 = call "Warten28"("Count(mSec)"=u32 100) -> ()  [unwired: 1 out]
            }
            frame #1 {
              n154 = global read "GVAIs.vi" "AIs"() -> (w1252:dbl[])
              n155 = Add(x=w1256, y=w1252) -> (x+y=w1255:dbl[])
              n156 = global read "GVTrapsMachs.vi" "Traps/Machs"() -> (w1251:dbl[])
              n157 = Add(x=w1251, y=w1254) -> (x+y=w1253:dbl[])
            }
          }
        }
        n158 = Divide(x=w1242, y=w1239) -> (x/y=w1241:dbl[])
        n159 = Divide(x=w1240, y=w1239) -> (x/y=w1238:dbl[])
        n160 = Build Array (concatenate)(w1241, w1238) -> (w1237:dbl[])
        n161 = global write "GVHK1Hz.vi" "Mod1Mod2Mod3/AITrapsMachs1Hz"(w1237) -> ()
      }
      n162 = while {
        tunnel: w439 -> [w856]
        tunnel: w508 -> [w855]
        tunnel: w507 -> [w854]
        tunnel: w506 -> [w853]
        shift-right: [w851] -> _
        shift-left: errorcluster {"status"=FALSE, "code"=0, "source"=""} ("error out") -> [w852]
        stop <- w857 stop-if-true
        n163 = call "AIsFIFORT-11-15.vi"("FPGA VI Reference In"=w856, "P2"=w855, "P1"=w854, "P0"=w853, "error in"=w852) -> ("error out"=w851:errorcluster)  [unwired: 1 in]
        "AIsFIFOread" <- w851
        n164 = global read "gvbooleschRT.vi" "global stop RT"() -> (w857:bool)
      }
      n165 = while {
        tunnel: w439 -> [w861]
        tunnel: w414 -> [w860]
        tunnel: w413 -> [w863]
        tunnel: w412 -> [w862]
        shift-right: [w858] -> _
        shift-left: errorcluster {"status"=FALSE, "code"=0, "source"=""} ("error out") -> [w859]
        stop <- w865 stop-if-true
        n166 = call "TrapsMachMitteln-11-15.vi"("FPGA VI Reference In"=w861, "Traps/MachKoeff2"=w860, "Traps/MachKoeff1"=w863, "Traps/MachKoeff0"=w862, "error in"=w859) -> ("error out"=w858:errorcluster)
        "MWTrapsMachs" <- w858
        n167 = call "Bis zum nächsten Vielfachen warten16"("Count(mSec)"=u32 100) -> ()  [unwired: 1 out]
        n168 = global read "gvbooleschRT.vi" "global stop RT"() -> (w865:bool)
      }
      n169 = while {
        shift-right: ["Methode"] -> _
        shift-left: w512 -> [w1259]
        stop <- w1261 stop-if-true
        n170 = call "Bis zum nächsten Vielfachen warten7"("Count(mSec)"=u32 1000) -> ()  [unwired: 1 out]
        n171 = global read "gvbooleschRT.vi" "global stop RT"() -> (w1261:bool)
        n172 = Not Equal?(x=w1259, y="Methode") -> (x != y?=w1257:bool)
        n173 = global write "GVMethodenwechsel.vi" "Methodenwechsel?"(w1257) -> ()
      }
      n174 = Add Array Elements(numeric array=w435) -> (sum=w434:i32)
      n175 = Array Size(array=w443) -> (size(s)=w464:i32)
      n176 = Unbundle(w460) -> ("created path"=w459:path, "created path"=w457:path, "created path"=w456:path, "Dateiname Housekeeping"=w458:string, "DateinameECD1"=w455:string, "DateinameECD2"=w454:string, "tdms0"=w453:refnum<k34>, "tdms1"=w452:refnum<k34>, "tdms0"=w451:refnum<k34>, "tdms1"=w450:refnum<k34>, "tdms0"=w449:refnum<k34>, "tdms1"=w448:refnum<k34>)
      n177 = Index Array(array=w436, index #1=0 ("Index"), index #2=1 ("Index"), index #3=2 ("Index"), index #4=3 ("Index")) -> (element #1=w475:i32, element #2=w474:i32, element #3=w477:i32, element #4=w476:i32)
      n178 = call <vilib>:"Space Constant.vi"() -> ("String"=w421:string)
      n179 = case shown="True" TRUE ("ECDSpeichern") {
        frame False {
        }
        frame True {
          w792 = errorcluster {"status"=FALSE, "code"=0, "source"=""} ("error out")
          w793 = dbl[] []
          n180 = global read "GVaktuelleTDMS.vi" "aktuelleTDMS-DateiECD1"() -> (w794:refnum<k34>)
          n181 = while {
            shift-right: [w806] -> _
            shift-left: w793 -> [w810]
            shift-right: [w799] -> _
            shift-left: w793 -> [w803]
            shift-right: [w805] -> _
            shift-left: w794 -> [w808]
            tunnel: w793 -> [w802]
            shift-right: [w796] -> _
            shift-left: w792 -> [w795]
            shift-right: [w798] -> _
            shift-left: w792 -> [w797]
            stop <- w815 stop-if-true
            n182 = call "Bis zum nächsten Vielfachen warten3"("Count(mSec)"=u32 500) -> ()  [unwired: 1 out]
            n183 = global read "GVECDs.vi" "ECD1MW"() -> (w809:dbl[])
            n184 = global read "GVECDs.vi" "ECD2MW"() -> (w800:dbl[])
            n185 = global read "gvbooleschRT.vi" "global stop RT"() -> (w815:bool)
            n186 = Build Array (concatenate)(w810, w809) -> (w807:dbl[])
            n187 = Build Array (concatenate)(w803, w800) -> (w804:dbl[])
            n188 = global read "GVaktuelleTDMS.vi" "aktuelleTDMS-DateiECD1"() -> (w805:refnum<k34>)
            n189 = global read "GVaktuelleTDMS.vi" "aktuelleTDMS-DateiECD2"() -> (w813:refnum<k34>)
            n190 = Equal?(x=w808, y=w805) -> (x = y?=w801:bool)
            n191 = TDMS Write(0:w805, 7:"ECD1", 9:w809, 11:w795) -> (15:w796:errorcluster)  [unwired: 2 in, 3 out]
            "TDMSwriteECD1" <- w796
            n192 = TDMS Write(0:w813, 7:"ECD2", 9:w800, 11:w797) -> (15:w798:errorcluster)  [unwired: 2 in, 3 out]
            "TDMSwriteECD2" <- w798
            n193 = Select(t=w807, s=w801, f=w802) -> (s? t:f=w806:dbl[])
            n194 = Select(t=w804, s=w801, f=w802) -> (s? t:f=w799:dbl[])
            n195 = global write "GVChroms.vi" "ECD1Chrom"(w806) -> ()
            n196 = global write "GVChroms.vi" "ECD2Chrom"(w799) -> ()
          }
        }
      }
      n197 = while {
        shift-right: [w520] -> _
        shift-left: w415 -> [w522]
        shift-right: [w519] -> _
        shift-left: w415 -> [w521]
        stop <- w524 stop-if-true
        n198 = call "Bis zum nächsten Vielfachen warten"("Count(mSec)"=u32 100) -> ()  [unwired: 1 out]
        n199 = case shown="True" "An/Aus" {
          tunnel: w522 -> [w526 w542]
          tunnel: w521 -> [w525 w541]
          tunnel: [w526 w535] -> w520
          tunnel: [w525 w534] -> w519
          frame False {
          }
          frame True {
            w538 = dbl[] [] ("t")
            n200 = global read "GVMWHorst.vi" "MWHorst"() -> (w531:dbl[])
            n201 = global read "GVTrapsMachs.vi" "Traps/Machs"() -> (w532:dbl[])
            n202 = Build Array (concatenate)(w532, w531) -> (w530:dbl[])
            n203 = Index Array(array=w530, index="dargestellte Größe 3") -> (element=w543:dbl)
            n204 = Build Array (concatenate)(w542, w543) -> (w536:dbl[])
            n205 = Select(t=w538, s="TafelWischen!", f=w536) -> (s? t:f=w535:dbl[])
            n206 = global read "GVZeitenZyklen.vi" "Big Ben, Methodenzeit, Zykluszeit0, Zykluszeit1, Zykluszeit2A, Zykluszeit2B"() -> (w529:dbl[])
            n207 = Index Array(array=w529, index=1 ("Index")) -> (element=w527:dbl)
            n208 = Build Array (concatenate)(w541, w527) -> (w537:dbl[])
            n209 = Select(t=w538, s="TafelWischen!", f=w537) -> (s? t:f=w534:dbl[])
            n210 = Bundle(w537, w536) -> (→"schnelleAnzeige":cluster{dbl[], dbl[]})  [unwired: 1 in]
          }
        }
        n211 = global read "gvbooleschRT.vi" "global stop RT"() -> (w524:bool)
      }
      n212 = case shown="True" TRUE ("HKSpeichern") {
        tunnel: w510 -> [_ w844]
        frame False {
        }
        frame True {
          n213 = while {
            tunnel: w844 -> [w848]
            shift-right: [w846] -> _
            shift-left: errorcluster {"status"=FALSE, "code"=0, "source"=""} ("error out") -> [w845]
            stop <- w850 stop-if-true
            n214 = call "Bis zum nächsten Vielfachen warten2"("Count(mSec)"=u32 1000) -> ()  [unwired: 1 out]
            n215 = local read "Methode"() -> (w847:i32)
            n216 = global read "gvbooleschRT.vi" "global stop RT"() -> (w850:bool)
            n217 = call "HKinTDMS-01-16.vi"("Methode"=w847, "error in (no error)"=w845, "Kanäle"=w848) -> ("error out"=w846:errorcluster)
            "TDMSwriteHK" <- w846
          }
        }
      }
      n218 = for {
        N: 1 -> [_]
        tunnel: w439 -> [w866]
        tunnel: [w866] -> w466
        n219 = call "Warten8"("Count(mSec)"=u32 100) -> ()  [unwired: 1 out]
      }
      n220 = global read "GVVentilposition.vi" "Ventilposition"() -> (w445:i32)
      n221 = Build Array(w421) -> (w420:string[])
      n222 = Initialize Array(-1 ("Element"), 4 ("Dimension")) -> (w437:i32[])
      n223 = case shown="True" TRUE {
        tunnel: w461 -> [_ w823]
        tunnel: w459 -> [_ w822]
        tunnel: w458 -> [_ w821]
        tunnel: w453 -> [_ w820]
        tunnel: w452 -> [_ w819]
        frame False {
        }
        frame True {
          w816 = errorcluster {"status"=FALSE, "code"=0, "source"=""} ("error out TDMSopen")
          n224 = while {
            shift-right: [w828] -> w818
            shift-left: w820 -> [w830]
            shift-right: [w839] -> w817
            shift-left: w819 -> [w832]
            shift-right: [w834] -> _
            shift-left: w823 -> [w840]
            tunnel: w821 -> [w836]
            tunnel: w822 -> [w837]
            shift-right: [w827] -> _
            shift-left: w816 -> [w825]
            shift-right: [w826] -> _
            shift-left: w816 -> [w824]
            stop <- w842 stop-if-true
            n225 = global read "GVZeitenZyklen.vi" "ZyklusNummernGesamt"() -> (w829:i32[])
            n226 = call "Bis zum nächsten Vielfachen warten5"("Count(mSec)"=u32 500) -> ()  [unwired: 1 out]
            n227 = Index Array(array=w829, index=1 ("Index")) -> (element=w834:i32)
            n228 = Greater?(x=w834, y=w840) -> (0:w833:bool)
            n229 = Select(t=w832, s=w833, f=w830) -> (s? t:f=w831:refnum<k34>)
            n230 = local read "Methode"() -> (w838:i32)
            n231 = global write "GVaktuelleTDMS.vi" "aktuelleTDMS-DateiHK"(w831) -> ()
            n232 = call "AktuelleTDMS.vi"("AktuelleTDMS"=w830, "error in TDMSopen"=w825, "Dateiordner"=w837, "NächsteTDMS"=w832, "NeuerZyklus?"=w833, "Methodennummer"=w838, "Zyklnumges"=w834, "error in TDMSclose"=w824, "Dateiname"=w836) -> ("AktuelleTDMS"=w828:refnum<k34>, "error out TDMSopen"=w827:errorcluster, "error out TDMSclose"=w826:errorcluster, "NächsteTDMS"=w839:refnum<k34>)  [unwired: 3 in]
            "TDMSopenHK" <- w827
            "TDMScloseHK" <- w826
            n233 = global read "gvbooleschRT.vi" "global stop RT"() -> (w842:bool)
          }
          n234 = TDMS Close(11:w818) -> ()  [unwired: 1 in, 2 out]
          n235 = TDMS Close(11:w817) -> ()  [unwired: 1 in, 2 out]
        }
      }
      n236 = case shown="True" TRUE {
        tunnel: w461 -> [_ w761]
        tunnel: w457 -> [_ w760]
        tunnel: w456 -> [_ w759]
        tunnel: w455 -> [_ w758]
        tunnel: w454 -> [_ w757]
        tunnel: w451 -> [_ w756]
        tunnel: w450 -> [_ w755]
        tunnel: w449 -> [_ w754]
        tunnel: w448 -> [_ w753]
        frame False {
        }
        frame True {
          n237 = while {
            shift-right: [w777] -> w752
            shift-left: w756 -> [w779]
            shift-right: [w787] -> w751
            shift-left: w755 -> [w781]
            shift-right: [w785] -> _
            shift-left: w761 -> [w788]
            tunnel: w760 -> [w784]
            tunnel: w758 -> [w783]
            stop <- w790 stop-if-true
            n238 = call "Bis zum nächsten Vielfachen warten4"("Count(mSec)"=u32 500) -> ()  [unwired: 1 out]
            n239 = local read "Methode"() -> (w786:i32)
            n240 = global read "gvbooleschRT.vi" "global stop RT"() -> (w790:bool)
            n241 = global read "GVZeitenZyklen.vi" "ZyklusNummernGesamt"() -> (w778:i32[])
            n242 = Index Array(array=w778, index=2 ("Index")) -> (element=w785:i32)
            n243 = Greater?(x=w785, y=w788) -> (0:w782:bool)
            n244 = Select(t=w781, s=w782, f=w779) -> (s? t:f=w780:refnum<k34>)
            n245 = global write "GVaktuelleTDMS.vi" "aktuelleTDMS-DateiECD1"(w780) -> ()
            n246 = call "AktuelleTDMS.vi"("AktuelleTDMS"=w779, "Dateiordner"=w784, "NächsteTDMS"=w781, "NeuerZyklus?"=w782, "Methodennummer"=w786, "Zyklnumges"=w785, "Dateiname"=w783) -> ("AktuelleTDMS"=w777:refnum<k34>, "NächsteTDMS"=w787:refnum<k34>)  [unwired: 5 in, 2 out]
          }
          n247 = while {
            shift-right: [w771] -> w750
            shift-left: w754 -> [w763]
            shift-right: [w772] -> w749
            shift-left: w753 -> [w765]
            shift-right: [w769] -> _
            shift-left: w761 -> [w773]
            tunnel: w759 -> [w768]
            tunnel: w757 -> [w767]
            stop <- w775 stop-if-true
            n248 = call "Bis zum nächsten Vielfachen warten6"("Count(mSec)"=u32 500) -> ()  [unwired: 1 out]
            n249 = local read "Methode"() -> (w770:i32)
            n250 = global read "gvbooleschRT.vi" "global stop RT"() -> (w775:bool)
            n251 = global read "GVZeitenZyklen.vi" "ZyklusNummernGesamt"() -> (w762:i32[])
            n252 = Index Array(array=w762, index=3 ("Index")) -> (element=w769:i32)
            n253 = Greater?(x=w769, y=w773) -> (0:w766:bool)
            n254 = Select(t=w765, s=w766, f=w763) -> (s? t:f=w764:refnum<k34>)
            n255 = global write "GVaktuelleTDMS.vi" "aktuelleTDMS-DateiECD2"(w764) -> ()
            n256 = call "AktuelleTDMS.vi"("AktuelleTDMS"=w763, "Dateiordner"=w768, "NächsteTDMS"=w765, "NeuerZyklus?"=w766, "Methodennummer"=w770, "Zyklnumges"=w769, "Dateiname"=w767) -> ("AktuelleTDMS"=w771:refnum<k34>, "NächsteTDMS"=w772:refnum<k34>)  [unwired: 5 in, 2 out]
          }
          n257 = TDMS Close(11:w752) -> ()  [unwired: 1 in, 2 out]
          n258 = TDMS Close(11:w751) -> ()  [unwired: 1 in, 2 out]
          n259 = TDMS Close(11:w750) -> ()  [unwired: 1 in, 2 out]
          n260 = TDMS Close(11:w749) -> ()  [unwired: 1 in, 2 out]
        }
      }
      n261 = Add(x=w477, y=w476) -> (x+y=w473:i32)
      n262 = Bundle(w420, w420, w420) -> (w484:cluster{string[], string[], string[]})  [unwired: 1 in]
      n263 = Index Array(array=w430, index=w428) -> (element=w429:T15)
      n264 = Initialize Array(cluster{"output high":dbl, "output low":dbl} {"output high"=99999.0, "output low"=0.0} ("output range"), w464) -> (w444:cluster{"output high":dbl, "output low":dbl}[])
      n265 = Concatenate Strings("?SE0,GDATA" ("Schreibpuffer"), "\r") -> (w416:string)
      n266 = Build Array(w475, w474, w473) -> (w472:i32[])
      n267 = while {
        tunnel: w511 -> [w990]
        shift-right: [w989] -> _
        shift-left: w430 -> [w971]
        tunnel: w444 -> [w988]
        tunnel: w443 -> [w987]
        tunnel: w439 -> [w986]
        tunnel: w442 -> [w985]
        tunnel: w441 -> [w984]
        shift-right: [w978] -> _
        shift-left: 0 -> [w983]
        tunnel: w439 -> [w982]
        tunnel: w438 -> [w981]
        shift-right: [w977] -> _
        shift-left: w437 -> [w980]
        tunnel: w436 -> [w972]
        tunnel: w435 -> [w973]
        tunnel: w434 -> [w974]
        tunnel: w433 -> [w975]
        tunnel: w432 -> [w976]
        tunnel: w431 -> [w979]
        shift-right: [w894] -> _
        shift-left: w429 -> [w893]
        tunnel: w414 -> [w872]
        tunnel: w413 -> [w876]
        tunnel: w412 -> [w882]
        i -> [w897]
        stop <- w991 stop-if-true
        w883 = 0  # ZeileMainMach2
        w884 = 0  # ZeileMainMach1
        w939 = FALSE
        w938 = 0.0
        w940 = 0  # ZeilennummerMPV
        w944 = cluster{dbl[], dbl[]} {[], []}
        w953 = dbl[] []
        w957 = 0  # ZeilePreMach2
        w958 = 0  # ZeilePreMach1
        w959 = 0  # ZeileFPGAFixp
        w960 = 0  # ZeileFPGAPID
        w961 = 0  # ZeileFPGABoolesch
        w962 = i32[] [0, 0, 0, 0]  # ZeilennummernHorst
        w963 = i32[] [0, 0, 0, 0]  # ZeilennummernDIOs
        n268 = Unbundle(w893) -> ("Zykluslängen [s]"=w937:dbl[], "ZeitpktDIOsMod0"=w936:dbl[], "ZeitpktDIOsMod1"=w935:dbl[], "ZeitpktDIOsMod2A"=w934:dbl[], "ZeitpktDIOsMod2B"=w933:dbl[], "DIOsSPMod0"=w932:bool[][], "DIOsSPMod1"=w931:bool[][], "DIOsSPMod2A"=w930:bool[][], "DIOsSPMod2B"=w929:bool[][], "Mod0HorstZeitpkt"=w928:dbl[], "Mod1HorstZeitpkt"=w927:dbl[], "Mod2AHorstZeitpkt"=w926:dbl[], "Mod2BHorstZeitpkt"=w925:dbl[], "HorstSPMod0"=w924:dbl[][], "HorstSPMod1"=w923:dbl[][], "HorstSPMod2A"=w922:dbl[][], "HorstSPMod2B"=w921:dbl[][], "LHSetpoints"=w920:dbl[], "LHHeizen?"=w919:bool[], "ZPktFPGABoolesch"=w918:dbl[], "FPGABoolesch"=w917:bool[][], "ZeitpktFPGAPID"=w916:dbl[], "FPGAPID"=w915:T17, "ZeitpktFPGAFixp"=w914:dbl[], "SHSetpoints"=w913:dbl[][], "t_PreMach1"=w912:dbl[], "T_PreMach1"=w911:dbl[], "t_PreMach2"=w910:dbl[], "T_PreMach2"=w909:dbl[], "PIDs für \"träge\" Heizungen"=w908:T18, "Zwangsbedingungen"=w907:dbl[][], "Dateien fürs MS schicken?"=w906:bool, "ZeitpunkteMPV"=w905:dbl[], "SPMPV"=w904:i32[], "ZeitpktMS-1"=w903:dbl, "ZeitpktMS-2"=w902:dbl, "Int.Start1"=w901:dbl, "Int.Stop1"=w900:dbl, "Int.Start2"=w899:dbl, "Int.Stop2"=w898:dbl, "t_MainMach1"=w892:dbl[], "T_MainMach1"=w891:dbl[], "t_MainMach2"=w890:dbl[], "T_MainMach2"=w889:dbl[])  [unwired: 1 out]
        n269 = Add(x=w980, y=1) -> (x+y=w948:i32[])
        n270 = Array Subset(array=w882, index=2 ("Index"), length=4 ("Länge")) -> (w879:dbl[])
        n271 = Array Subset(array=w876, index=2 ("Index"), length=4 ("Länge")) -> (w875:dbl[])
        n272 = Array Subset(array=w872, index=2 ("Index"), length=4 ("Länge")) -> (w871:dbl[])
        n273 = local read "Methode"() -> (w896:i32)
        n274 = while {
          tunnel: w973 -> [w1064]
          tunnel: w976 -> [w1062]
          tunnel: w975 -> [w1061]
          tunnel: w972 -> [w1063]
          tunnel: w974 -> [w1060]
          tunnel: w907 -> [w1053]
          stop <- w1054 stop-if-true
          n275 = shared-variable "NI-cRIO9022-0150923B\\CRIOVariablen.lvlib\\STOPP!"() -> (w1050:bool)  [unwired: 1 in, 1 out]
          n276 = call "Bis zum nächsten Vielfachen warten10"("Count(mSec)"=u32 1000) -> ()  [unwired: 1 out]
          n277 = local read "Methode"() -> (w1059:i32)
          n278 = Or(x="global stop RT", y=w1050) -> (x .or. y?=w1051:bool)
          n279 = global read "GVMethodenwechsel.vi" "Methodenwechsel?"() -> (w1056:bool)
          n280 = global read "gvbooleschRT.vi" "global stop RT"() -> (w1057:bool)
          n281 = case shown="True" w1051 {
            frame False {
            }
            frame True {
              n282 = global write "gvbooleschRT.vi" "global stop RT"(TRUE ("global stop RT")) -> ()
            }
          }
          n283 = call "ZwangsbedingungenGV.vi"("AnzahlHorst"=w1062, "AnzahlHorst/Modul"=w1063, "AnzahlLH"=w1061, "AnzahlDIOs/Modul"=w1064, "AnzahlDIOs"=w1060, "Zwangsbedingungen"=w1053, "Methodennummer"=w1059) -> ("Methodennummer"=w1058:i32)  [unwired: 4 in]
          n284 = local write "Methode"(w1058) -> ()
          n285 = local read "veränderte Methode benutzen"() -> (w1055:bool)
          n286 = Compound Arithmetic op=OR(w1057, w1056, w1055) -> (w1054:bool)
        }
        n287 = while {
          tunnel: w987 -> [w1047]
          tunnel: w988 -> [w1048]
          tunnel: w986 -> [w1046]
          tunnel: w920 -> [w1045]
          tunnel: w908 -> [w1044]
          stop <- w1040 stop-if-true
          n288 = call "LH-01-16.vi"("PIDs für \"träge\" Heizungen"=w1044, "AIsLH"=w1047, "LHSetpoints"=w1045, "OutputRange"=w1048, "FPGA VI Reference In"=w1046) -> ()
          n289 = call "Bis zum nächsten Vielfachen warten12"("Count(mSec)"=u32 100) -> ()  [unwired: 1 out]
          n290 = global read "GVMethodenwechsel.vi" "Methodenwechsel?"() -> (w1042:bool)
          n291 = global read "gvbooleschRT.vi" "global stop RT"() -> (w1043:bool)
          n292 = local read "veränderte Methode benutzen"() -> (w1041:bool)
          n293 = Compound Arithmetic op=OR(w1043, w1042, w1041) -> (w1040:bool)
        }
        n294 = Build Cluster Array(w932, w931, w930, w929) -> (w967:cluster{"DIOsSPMod2B":bool[][]}[])
        n295 = Build Cluster Array(w924, w923, w922, w921) -> (w965:cluster{"HorstSPMod2B":dbl[][]}[])
        n296 = Build Cluster Array(w936, w935, w934, w933) -> (w968:cluster{"ZeitpktDIOsMod2B":dbl[]}[])
        n297 = Build Cluster Array(w928, w927, w926, w925) -> (w966:cluster{"Mod2BHorstZeitpkt":dbl[]}[])
        n298 = Bundle(w879, w875, w871) -> (w870:cluster{dbl[], dbl[], dbl[]})  [unwired: 1 in]
        n299 = Equal?(x=w897, y=0) -> (x = y?=w969:bool)
        n300 = global read "GVZeitenZyklen.vi" "ZyklusNummern"() -> (w947:i32[])
        n301 = global read "GVZwangs.vi" "ZwangsHorst?"() -> (w952:cluster{bool[]}[])
        n302 = global read "gvbooleschRT.vi" "global stop RT"() -> (w991:bool)
        n303 = global read "GVZwangsMPV.vi" "ZwangsMPV?"() -> (w868:bool)
        n304 = global read "GVZwangs.vi" "ZwangsDIO?"() -> (w951:cluster{bool[]}[])
        n305 = global read "GVaktuelleTDMS.vi" "aktuelleTDMS-DateiECD1"() -> (w946:refnum<k34>)
        n306 = global read "GVZwangs.vi" "ZwangsFPGABoolesch?"() -> (w950:bool[])
        n307 = while {
          shift-right: [w1004] -> _
          shift-left: w939 -> [w1008]
          shift-right: [w1003] -> _
          shift-left: w938 -> [w1007]
          shift-right: [w1002] -> _
          shift-left: w939 -> [w1006]
          shift-right: [w1001] -> _
          shift-left: w938 -> [w1005]
          tunnel: w979 -> [w1000]
          tunnel: w901 -> [w995]
          tunnel: w900 -> [w994]
          tunnel: w899 -> [w993]
          tunnel: w898 -> [w992]
          stop <- w997 stop-if-true
          n308 = call "Integrieren.vi"("Integrieren1"=w1008, "Integral1"=w1007, "Integrieren2"=w1006, "Integral2"=w1005, "Int.Start1"=w995, "Int.Stop1"=w994, "Int.Start2"=w993, "HorstProbenflußNr."=w1000, "Int.Stop2"=w992) -> ("Integrieren1"=w1004:bool, "Integral1"=w1003:dbl, "Integrieren2"=w1002:bool, "Integral2"=w1001:dbl)  [unwired: 7 in]
          n309 = call "Bis zum nächsten Vielfachen warten9"("Count(mSec)"=u32 100) -> ()  [unwired: 1 out]
          n310 = global read "GVMethodenwechsel.vi" "Methodenwechsel?"() -> (w998:bool)
          n311 = global read "gvbooleschRT.vi" "global stop RT"() -> (w999:bool)
          n312 = local read "veränderte Methode benutzen"() -> (w996:bool)
          n313 = Compound Arithmetic op=OR(w999, w998, w996) -> (w997:bool)
        }
        n314 = while "Zeit" {
          tunnel: w969 -> [w1196]
          tunnel: w937 -> [w1194]
          tunnel: w948 -> [w1189]
          tunnel: [w1188] -> w977
          shift-right: [w1185] -> _
          shift-left: 0.0 -> [w1186]
          i -> [w1198]
          stop <- w1191 stop-if-true
          n315 = Equal?(x=w1198, y=0) -> (x = y?=w1187:bool)
          n316 = call "Bis zum nächsten Vielfachen warten15"("Count(mSec)"=u32 50) -> ()  [unwired: 1 out]
          n317 = call "BigBen-01-16.vi"("MethodenStartzeit"=w1186, "Methodenstart?"=w1187, "Programmstart?"=w1196, "Zykluslängen [s]"=w1194, "MethodenStartZyklusNummern"=w1189) -> ("MethodenStartzeit"=w1185:dbl, "ZyklusNummernGesamt"=w1188:i32[])  [unwired: 2 in]
          n318 = global read "GVMethodenwechsel.vi" "Methodenwechsel?"() -> (w1190:bool)
          n319 = global read "gvbooleschRT.vi" "global stop RT"() -> (w1195:bool)
          n320 = local read "veränderte Methode benutzen"() -> (w1193:bool)
          n321 = Or(x=w1190, y=w1195) -> (x .or. y?=w1192:bool)
          n322 = Or(x=w1193, y=w1192) -> (x .or. y?=w1191:bool)
        }
        n323 = Bundle(w968, w967, w966, w965, "LHHeizen?"=w919, "ZPktFPGABoolesch"=w918, "FPGABoolesch"=w917, "ZeitpktFPGAPID"=w916, "FPGAPID"=w915, "ZeitpktFPGAFixp"=w914, "SHSetpoints"=w913, "t_PreMach1"=w912, "T_PreMach1"=w911, "t_PreMach2"=w910, "T_PreMach2"=w909, "ZeitpunkteMPV"=w905, "SPMPV"=w904, "t_MainMach1"=w892, "T_MainMach1"=w891, "t_MainMach2"=w890, "T_MainMach2"=w889) -> (w964:T19)  [unwired: 1 in]
        n324 = Index Array(array=w971, index=w896) -> (element=w895:T15)
        n325 = while {
          tunnel: w990 -> [w1211]
          shift-right: [w1202] -> _
          shift-left: w895 -> [w1210]
          tunnel: w896 -> [w1208]
          shift-right: [w1200] -> w989
          shift-left: w971 -> [w1209]
          tunnel: [w1201] -> w894
          stop <- w1204 stop-if-true
          n326 = call "Bis zum nächsten Vielfachen warten8"("Count(mSec)"=u32 500) -> ()  [unwired: 1 out]
          n327 = global read "GVMethodenwechsel.vi" "Methodenwechsel?"() -> (w1206:bool)
          n328 = global read "gvbooleschRT.vi" "global stop RT"() -> (w1205:bool)
          n329 = case shown="True" "Methode verändern" {
            tunnel: w1211 -> [_ w1233]
            tunnel: w1210 -> [w1230 w1232]
            tunnel: [w1230 w1231] -> w1202
            frame False {
            }
            frame True {
              n330 = call "methodeändern-11-15.vi"("Methode"=w1232, "Namen"=w1233) -> ("Methode"=w1231:T20)  [unwired: 1 in]
              n331 = property on="Methode verändern" class="Bool (strict)"("Value"=FALSE ("Methode verändern")) -> ()  [unwired: 2 in, 2 out]
            }
          }
          n332 = Compound Arithmetic op=OR(w1206, w1205, "veränderte Methode benutzen") -> (w1204:bool)
          n333 = case shown="True" "Methode speichern" {
            tunnel: w1202 -> [_ w1227]
            tunnel: w1209 -> [w1220 w1229]
            tunnel: w1208 -> [_ w1228]
            tunnel: [w1220 w1222] -> w1200
            frame False {
            }
            frame True {
              n334 = Replace Array Subset(array=w1229, new element=w1227, index=w1228) -> (w1222:T9)
              n335 = property on="Methode speichern" class="Bool (strict)"("Value"=FALSE ("Methode speichern")) -> ()  [unwired: 2 in, 2 out]
              n336 = Open/Create/Replace File(file path (use dialog)=path "c:/methoden.per" ("Dateipfad (Dialog verwenden)"), operation (0:open)=T10."replace" ("Operation (0:Öffnen)")) -> (refnum out=w1224:refnum<file>)  [unwired: 4 in, 2 out]
              n337 = Write to Binary File(file (use dialog)=w1224, data=w1222) -> (refnum out=w1221:refnum<file>)  [unwired: 4 in, 2 out]
              n338 = Close File(refnum=w1221) -> ()  [unwired: 1 in, 2 out]
            }
          }
          n339 = case shown="False" "veränderte Methode benutzen" {
            tunnel: w1202 -> [_ w1217]
            tunnel: [w1214 w1217] -> w1201
            tunnel: w1200 -> [w1216 _]
            frame False {
              n340 = local read "Methode"() -> (w1215:i32)
              n341 = Index Array(array=w1216, index=w1215) -> (element=w1214:T15)
            }
            frame True {
              n342 = flat-sequence {
                frame #0 {
                  n343 = call "Warten"("Count(mSec)"=u32 1100) -> ()  [unwired: 1 out]
                }
                frame #1 {
                  n344 = property on="veränderte Methode benutzen" class="Bool (strict)"("Value"=FALSE ("Methode verändern")) -> ()  [unwired: 2 in, 2 out]
                }
              }
            }
          }
        }
        n345 = Bundle(w953, w953, w953, w953) -> (w954:cluster{dbl[], dbl[], dbl[], dbl[]})  [unwired: 1 in]
        n346 = Bundle("ZyklusNummern"=w947, "ZeilennummernDIOs"=w963, "ZwangsDIO?"=w951, "ZeilennummernHorst"=w962, "ZwangsHorst?"=w952, "ZeileFPGABoolesch"=w961, "ZwangsFPGABoolesch?"=w950, "ZeileFPGAPID"=w960, "ZeileFPGAFixp"=w959, "ZeilePreMach1"=w958, "ZeilePreMach2"=w957, "ZeilennummerMPV"=w940, "ZeileMainMach1"=w884, "ZeileMainMach2"=w883, "ZwangsMPV?"=w868) -> (w956:T21)  [unwired: 1 in]
        n347 = call "arrayDoppelMoppel-11-15.vi"("verdoppeln"=i32[] [0, 1], "Traps/MachsKoeff2"=w872, "Traps/MachsKoeff1"=w876, "Traps/MachsKoeff0"=w882) -> ("Traps/MachsKoeff2"=w885:dbl[], "Traps/MachsKoeff1"=w886:dbl[], "Traps/MachsKoeff0"=w887:dbl[])  [unwired: 5 in]
        n348 = while "ZyklusSteuerung" {
          tunnel: w981 -> [w1183]
          tunnel: w982 -> [w1176]
          shift-right: [w1172] -> _
          shift-left: w956 -> [w1181]
          tunnel: w964 -> [w1182]
          tunnel: w887 -> [w1175]
          tunnel: w886 -> [w1174]
          tunnel: w885 -> [w1173]
          tunnel: w870 -> [w1171]
          stop <- w1177 stop-if-true
          n349 = call "ZyklussteuerungGV-11-15.vi"("Traps/MachKoeff0"=w1175, "DIOsNummern"=w1183, "FPGA VI Reference In"=w1176, "Traps/MachKoeff1"=w1174, "ServosWarmHigh (us)KaltHigh(us)"="ServosWarmHigh (us)KaltHigh(us)", "Traps/MachKoeff2"=w1173, "Schieberegister"=w1181, "Zeitpunkte/Setpoints"=w1182, "MachKoeffs"=w1171) -> ("Schieberegister"=w1172:T22)  [unwired: 6 in]
          n350 = call "Bis zum nächsten Vielfachen warten11"("Count(mSec)"=u32 100) -> ()  [unwired: 1 out]
          n351 = global read "GVMethodenwechsel.vi" "Methodenwechsel?"() -> (w1180:bool)
          n352 = global read "gvbooleschRT.vi" "global stop RT"() -> (w1179:bool)
          n353 = local read "veränderte Methode benutzen"() -> (w1178:bool)
          n354 = Compound Arithmetic op=OR(w1180, w1179, w1178) -> (w1177:bool)
        }
        n355 = while {
          shift-right: [w1118] -> _
          shift-left: w954 -> [w1125]
          shift-right: [w1117] -> _
          shift-left: w954 -> [w1124]
          shift-right: [w1115] -> _
          shift-left: T13 {"Zyklus1"=0, "Zeitachse1"=0, "dargestellte Größe 1"=0, "Zyklus2"=0, "Zeitachse2"=0, "dargestellte Größe 2"=0} ("AnzeigeEinstellungen") -> [w1123]
          tunnel: w937 -> [w1093]
          shift-right: [w1089] -> _
          shift-left: w946 -> [w1088]
          shift-right: [w1084] -> _
          shift-left: w944 -> [w1086]
          shift-right: [w1074] -> _
          shift-left: w944 -> [w1085]
          shift-right: ["Detektor"] -> _
          shift-left: 0 ("Detektor") -> [w1082]
          stop <- w1129 stop-if-true
          w1094 = 0.0 ("X-Achse.Bereich:Minimum")
          n356 = call "Bis zum nächsten Vielfachen warten14"("Count(mSec)"=u32 1000) -> ()  [unwired: 1 out]
          n357 = global read "GVMWHorst.vi" "MWHorst"() -> (→"MWHorst":dbl[])
          n358 = case shown="True" TRUE ("Tabellarische Darstellung") {
            frame False {
            }
            frame True {
              n359 = global read "GVHK1Hz.vi" "Mod1Mod2Mod3/AITrapsMachs1Hz"() -> (w1135:dbl[])
              n360 = Array Subset(array=w1135, index=0 ("Index"), length=32 ("Länge")) -> (→"AIs1":dbl[])
              n361 = Array Subset(array=w1135, index=32 ("Index"), length=32 ("Länge")) -> (→"AIs2":dbl[])
              n362 = Array Subset(array=w1135, index=64 ("Index"), length=32 ("Länge")) -> (→"AIs3":dbl[])
            }
          }
          n363 = case shown="0, Default" "Detektor" {
            tunnel: [w1149 w1161] -> w1084
            tunnel: w1093 -> [w1148 w1163]
            tunnel: "Detektor" -> [w1143 w1157]
            tunnel: [w1147 w1162] -> w1091
            tunnel: [w1146 w1160] -> w1089
            frame 0, Default {
              n364 = Increment(x=w1143) -> (x+1=w1144:i32)
              n365 = Increment(x=w1144) -> (x+1=w1142:i32)
              n366 = global read "GVChroms.vi" "ECD1Chrom"() -> (w1145:dbl[])
              n367 = global read "GVaktuelleTDMS.vi" "aktuelleTDMS-DateiECD1"() -> (w1146:refnum<k34>)
              n368 = Index Array(array=w1148, index=w1142) -> (element=w1147:dbl)
              n369 = Array Size(array=w1145) -> (size(s)=w1151:i32)
              n370 = for {
                N: w1151 -> [_]
                tunnel: [w1152] -> w1150 mode=indexing
                i -> [w1155]
                n371 = To Double Precision Float(number=w1155) -> (double precision float=w1154:dbl)
                n372 = Divide(x=w1154, y=10.0) -> (x/y=w1152:dbl)
              }
              n373 = Bundle(w1150, "ECD1Chrom"=w1145) -> (w1149:cluster{dbl[], "ECD1Chrom":dbl[]})  [unwired: 1 in]
            }
            frame 1 {
              n374 = Increment(x=w1157) -> (x+1=w1158:i32)
              n375 = Increment(x=w1158) -> (x+1=w1156:i32)
              n376 = global read "GVChroms.vi" "ECD2Chrom"() -> (w1159:dbl[])
              n377 = global read "GVaktuelleTDMS.vi" "aktuelleTDMS-DateiECD2"() -> (w1160:refnum<k34>)
              n378 = Index Array(array=w1163, index=w1156) -> (element=w1162:dbl)
              n379 = Array Size(array=w1159) -> (size(s)=w1165:i32)
              n380 = for {
                N: w1165 -> [_]
                tunnel: [w1166] -> w1164 mode=indexing
                i -> [w1169]
                n381 = To Double Precision Float(number=w1169) -> (double precision float=w1168:dbl)
                n382 = Divide(x=w1168, y=10.0) -> (x/y=w1166:dbl)
              }
              n383 = Bundle(w1164, "ECD2Chrom"=w1159) -> (w1161:cluster{dbl[], "ECD2Chrom":dbl[]})  [unwired: 1 in]
            }
          }
          n384 = Equal?(x="Detektor", y=w1082) -> (x = y?=w1081:bool)
          n385 = Subtract(x="HK1YMax", y="HK1YMin") -> (x-y=w1109:dbl)
          n386 = Subtract(x="HK2YMax", y="HK2YMin") -> (x-y=w1104:dbl)
          n387 = Subtract(x="DetYMax", y="DetYMin") -> (x-y=w1099:dbl)
          n388 = global read "GVMethodenwechsel.vi" "Methodenwechsel?"() -> (w1127:bool)
          n389 = global read "GVZeitenZyklen.vi" "ZyklusNummern"() -> (w1096:i32[])
          "ZyklusNummern" <- w1096
          n390 = global read "GVMetavariablen.vi" "Metavariablen"() -> (→"Metavariablen":dbl[])
          n391 = global read "gvbooleschRT.vi" "global stop RT"() -> (w1128:bool)
          n392 = global read "GVVentilposition.vi" "Ventilposition"() -> (→"Ventilposition":i32)
          n393 = Divide(x=w1109, y=10.0) -> (x/y=w1107:dbl)
          n394 = Divide(x=w1104, y=10.0) -> (x/y=w1102:dbl)
          n395 = Divide(x=w1099, y=20.0) -> (x/y=w1097:dbl)
          n396 = global read "GVZeitenZyklen.vi" "ZyklusNummernGesamt"() -> (→"ZyklusNummernGesamt":i32[])
          n397 = local read "veränderte Methode benutzen"() -> (w1126:bool)
          n398 = Or(x=w1127, y=w1128) -> (x .or. y?=w1130:bool)
          n399 = global read "GVZeitenZyklen.vi" "Big Ben, Methodenzeit, Zykluszeit0, Zykluszeit1, Zykluszeit2A, Zykluszeit2B"() -> (w1069:dbl[])
          n400 = Or(x=w1130, y=w1126) -> (x .or. y?=w1129:bool)
          n401 = Index Array(array=w1069, index=0) -> (element=w1067:dbl)
          n402 = To Long Integer(number=w1069) -> (32bit integer=→"Big Ben, Methodenzeit, Zykluszeit0, Zykluszeit1, Zykluszeit2A, Zykluszeit2B":i32[])
          n403 = shared-variable "NI-cRIO9022-0150923B\\CRIOVariablen.lvlib\\BigBen"(w1067) -> ()  [unwired: 1 in, 1 out]
          n404 = Equal?(x=w1089, y=w1088) -> (x = y?=w1087:bool)
          n405 = call "AnzeigeGV.vi"("veränderte Methode benutzen"=w1126, "Zykluslängen [s]"=w1093, "Cluster1"=w1125, "Big Ben, Methodenzeit, Zykluszeit0, Zykluszeit1, Zykluszeit2A, Zykluszeit2B"=w1069, "Zyklusnummern 0, 1, 2A, 2B"=w1096, "Cluster2"=w1124, "AnzeigeEinstellungen"=w1123, "dargestellte Größe 1"="dargestellte Größe 1", "Zeitachse1"="Zeitachse1", "dargestellte Größe 2"="dargestellte Größe 2", "Zeitachse2"="Zeitachse2") -> ("Anzeige2"=→"Housekeeping2":cluster{dbl[], dbl[]}, "Cluster1"=w1118:cluster{dbl[], dbl[], dbl[], dbl[]}, "x1Inkr"=w1113:dbl, "Cluster2"=w1117:cluster{dbl[], dbl[], dbl[], dbl[]}, "Anzeige1"=→"Housekeeping1":cluster{dbl[], dbl[]}, "AnzeigeEinstellungen"=w1115:T13, "x2Max"=w1077:dbl, "x2Inkr"=w1112:dbl, "x1Max"=w1078:dbl)  [unwired: 8 in]
          n406 = Divide(x=w1091, y=20.0) -> (x/y=w1092:dbl)
          n407 = Select(t=w1085, s=w1087, f=w1086) -> (s? t:f=w1080:cluster{dbl[], dbl[]})
          n408 = property on="Housekeeping1" class="XYGraph (strict)"("XScale.Minimum"=w1094, "XScale.Maximum"=w1078, "XScale.Increment"=w1113, "YScale.Minimum"="HK1YMin", "YScale.Maximum"="HK1YMax", "YScale.Increment"=w1107) -> ()  [unwired: 2 in, 2 out]
          n409 = property on="Housekeeping2" class="XYGraph (strict)"("XScale.Minimum"=w1094, "XScale.Maximum"=w1077, "XScale.Increment"=w1112, "YScale.Minimum"="HK2YMin", "YScale.Maximum"="HK2YMax", "YScale.Increment"=w1102) -> ()  [unwired: 2 in, 2 out]
          n410 = property on="Detektor 2" class="XYGraph (strict)"("XScale.Minimum"=w1094, "XScale.Maximum"=w1091, "XScale.Increment"=w1092, "YScale.Minimum"="DetYMin", "YScale.Maximum"="DetYMax", "YScale.Increment"=w1097) -> ()  [unwired: 2 in, 2 out]
          n411 = Select(t=w1080, s=w1081, f=cluster{dbl[], dbl[]} {[], []} ("s? t:f")) -> (s? t:f=w1074:cluster{dbl[], dbl[]})
          n412 = Build Array(w1084, w1074) -> (→"Detektor 2":cluster{dbl[], "ECD2Chrom":dbl[]}[])
        }
        n413 = global read "GVZeitenZyklen.vi" "Big Ben, Methodenzeit, Zykluszeit0, Zykluszeit1, Zykluszeit2A, Zykluszeit2B"() -> (w943:dbl[])
        n414 = Index Array(array=w943, index=3 ("Index")) -> (element=w941:dbl)
        n415 = while {
          tunnel: w985 -> [w1012]
          tunnel: w984 -> [w1011]
          tunnel: w906 -> [w1026]
          shift-right: [w1027] -> w978
          shift-left: w983 -> [w1028]
          tunnel: w903 -> [w1022]
          tunnel: w902 -> [w1016]
          shift-right: [w1013] -> _
          shift-left: w941 -> [w1017]
          stop <- w1029 stop-if-true
          n416 = Less?(x=w1017, y=w1022) -> (x < y?=w1020:bool)
          n417 = Less?(x=w1017, y=w1016) -> (x < y?=w1018:bool)
          n418 = call "Bis zum nächsten Vielfachen warten13"("Count(mSec)"=u32 100 ("Zu wartende ms")) -> ()  [unwired: 1 out]
          n419 = global read "GVMethodenwechsel.vi" "Methodenwechsel?"() -> (w1031:bool)
          n420 = global read "gvbooleschRT.vi" "global stop RT"() -> (w1032:bool)
          n421 = local read "veränderte Methode benutzen"() -> (w1030:bool)
          n422 = global read "GVZeitenZyklen.vi" "Big Ben, Methodenzeit, Zykluszeit0, Zykluszeit1, Zykluszeit2A, Zykluszeit2B"() -> (w1024:dbl[])
          n423 = Compound Arithmetic op=OR(w1032, w1031, w1030) -> (w1029:bool)
          n424 = Index Array(array=w1024, index=3 ("Index")) -> (element=w1013:dbl)
          n425 = Greater Or Equal?(x=w1013, y=w1022) -> (x >= y?=w1021:bool)
          n426 = Greater Or Equal?(x=w1013, y=w1016) -> (x >= y?=w1019:bool)
          n427 = And(x=w1019, y=w1018) -> (x .and. y?=w1015:bool)
          n428 = And(x=w1021, y=w1020) -> (x .and. y?=w1010:bool)
          n429 = Or(x=w1010, y=w1015) -> (x .or. y?=w1014:bool)
          n430 = And(x=w1026, y=w1014) -> (x .and. y?=w1025:bool)
          n431 = case shown="True" w1025 {
            tunnel: w1028 -> [w1034 w1035]
            tunnel: [w1034 w1039] -> w1027
            tunnel: w1012 -> [_ w1038]
            tunnel: w1011 -> [_ w1037]
            tunnel: w1010 -> [_ w1036]
            frame False {
            }
            frame True {
              n432 = call "MSDateienSchicken12-15.vi"("MSNummer"=w1035, "MSa?"=w1036, "Dateipfad:fromcriordy"=w1037, "Dateipfad:fromcriocmd"=w1038) -> ()  [unwired: 1 in]
              n433 = Increment(x=w1035) -> (x+1=w1039:i32)
            }
          }
        }
      }
      n434 = Add Array Elements(numeric array=w472) -> (sum=w482:i32)
      n435 = Index Array(array=w472, index #1=0 ("Index"), index #2=1 ("Index")) -> (element #1=w493:i32, element #2=w491:i32)
      n436 = Split 1D Array(array=w471, index=w493) -> (first subarray=w497:dbl[], second subarray=w501:dbl[])
      n437 = Split 1D Array(array=w469, index=w493) -> (first subarray=w500:string[], second subarray=w502:string[])
      n438 = Split 1D Array(array=w470, index=w493) -> (first subarray=w490:string[], second subarray=w492:string[])
      n439 = Initialize Array(-1.0 ("Element"), w482) -> (w467:dbl[])
      n440 = Split 1D Array(array=w502, index=w491) -> (first subarray=w499:string[], second subarray=w498:string[])
      n441 = Split 1D Array(array=w501, index=w491) -> (first subarray=w496:dbl[], second subarray=w495:dbl[])
      n442 = Split 1D Array(array=w492, index=w491) -> (first subarray=w489:string[], second subarray=w488:string[])
      n443 = Bundle(w500, w499, w498, w497, w496, w495) -> (w494:T23)  [unwired: 1 in]
      n444 = Bundle(w490, w489, w488) -> (w487:cluster{string[], string[], string[]})  [unwired: 1 in]
      n445 = Initialize Array(0.0, 8 ("Dimension")) -> (w417:dbl[])
      n446 = Bundle(w486, w486, w486) -> (w485:cluster{i32, i32, i32})  [unwired: 1 in]
      n447 = Initialize Array("x", 8 ("Dimension")) -> (w422:string[])
      n448 = case shown="True" TRUE ("SerielleKomm.") {
        tunnel: bool[] [TRUE, TRUE, TRUE, TRUE, TRUE, TRUE, TRUE, TRUE] -> [_ w560]
        tunnel: w422 -> [_ w559]
        tunnel: w494 -> [_ w558]
        tunnel: w493 -> [_ w557]
        tunnel: w491 -> [_ w556]
        tunnel: w487 -> [_ w555]
        tunnel: w485 -> [_ w554]
        tunnel: w484 -> [_ w553]
        tunnel: w471 -> [_ w552]
        tunnel: w468 -> [_ w551]
        tunnel: w467 -> [_ w550]
        tunnel: w466 -> [_ w547]
        tunnel: w445 -> [_ w549]
        tunnel: w417 -> [_ w548]
        tunnel: w416 -> [_ w546]
        frame False {
        }
        frame True {
          n449 = while {
            tunnel: w547 -> [w571]
            tunnel: w546 -> [w564]
            shift-right: [w561] -> _
            shift-left: errorcluster {"status"=FALSE, "code"=0, "source"=""} ("error out") -> [w563]
            stop <- w573 stop-if-true
            n450 = String To Byte Array(string=w564) -> (unsigned byte array=w567:u8[])
            n451 = call "Warten6"("Count(mSec)"=u32 500) -> ()  [unwired: 1 out]
            n452 = Join Numbers(hi=w567, lo=u8 5) -> ((hi.lo)=w569:u16[])
            n453 = Join Numbers(hi=w567, lo=u8 6) -> ((hi.lo)=w565:u16[])
            n454 = xnode "Invoke Method"("FPGA VI Reference In"=w571, "error in"=w563, "Data"=w569) -> ("FPGA VI Reference Out"=w568:refnum<k20>, "error out"=w562:errorcluster)  [unwired: 1 in, 1 out]
            n455 = global read "gvbooleschRT.vi" "global stop RT"() -> (w573:bool)
            n456 = xnode "Invoke Method"("FPGA VI Reference In"=w568, "error in"=w562, "Data"=w565) -> ("error out"=w561:errorcluster)  [unwired: 1 in, 2 out]
            "writeFIFORS485" <- w561
          }
          n457 = while {
            shift-right: [w737] -> _
            shift-left: w560 -> [w712]
            shift-right: [w720] -> _
            shift-left: w550 -> [w732]
            tunnel: w547 -> [w719]
            shift-right: [w710] -> _
            shift-left: w559 -> [w736]
            tunnel: w551 -> [w735]
            tunnel: w552 -> [w734]
            shift-right: [w722] -> _
            shift-left: w553 -> [w724]
            tunnel: w557 -> [w730]
            tunnel: w556 -> [w731]
            tunnel: w558 -> [w733]
            tunnel: w555 -> [w727]
            shift-right: [w726] -> _
            shift-left: w554 -> [w728]
            shift-right: [w716] -> _
            shift-left: w549 -> [w718]
            shift-right: [w713] -> _
            shift-left: w548 -> [w714]
            shift-right: [w706] -> _
            shift-left: errorcluster {"status"=FALSE, "code"=0, "source"=""} ("error out") -> [w709]
            stop <- w721 stop-if-true
            n458 = for {
              tunnel: w712 -> [w741] mode=indexing
              tunnel: w714 -> [w738] mode=indexing
              tunnel: [w745] -> w713 mode=indexing
              tunnel: [w742] -> w711 mode=indexing
              n459 = global read "GVZeitenZyklen.vi" "Big Ben, Methodenzeit, Zykluszeit0, Zykluszeit1, Zykluszeit2A, Zykluszeit2B"() -> (w748:dbl[])
              n460 = Index Array(array=w748, index=0 ("Index")) -> (element=w746:dbl)
              n461 = Subtract(x=w746, y=w738) -> (x-y=w744:dbl)
              n462 = Greater?(x=w744, y=0.1) -> (0:w740:bool)
              n463 = Or(x=w741, y=w740) -> (x .or. y?=w739:bool)
              n464 = Select(t=w740, s=w740, f=w741) -> (s? t:f=w742:bool)
              n465 = Select(t=w746, s=w739, f=w738) -> (s? t:f=w745:dbl)
            }
            n466 = call "MPVSenden-11-15.vi"("Ventilposition"=w718, "error in"=w709, "FPGA VI Reference In"=w719) -> ("Ventilposition"=w716:i32, "error out"=w708:errorcluster, "FPGA VI Reference Out"=w717:refnum<k20>)
            n467 = call "Warten3"("Count(mSec)"=u32 50) -> ()  [unwired: 1 out]
            n468 = global read "GVHorstSP.vi" "HorstSP"() -> (w720:dbl[])
            n469 = Not Equal?(x=w720, y=w732) -> (x != y?=w725:bool)
            n470 = global read "gvbooleschRT.vi" "global stop RT"() -> (w721:bool)
            n471 = call "NeueSP.vi"("Anzahl2"=w731, "Anzahl1"=w730, "AlteSP"=w732, 7:"NeueSP"=w720, "BefehleCluster"=w724, 10:"NeueSP"=w725, "ClusterFest"=w733) -> ("BefehleCluster"=w723:T24)  [unwired: 4 in]
            n472 = call "Senden-11-15.vi"("BefehlsCluster"=w723, "error in"=w708, "AbfragenCluster"=w727, "Abfragenr.Cluster"=w728, "Senden?"=w711, "FPGA VI Reference In"=w717) -> ("BefehlsCluster"=w722:T24, "error out"=w707:errorcluster, "Senden?"=w729:bool[], "Abfragenr.Cluster"=w726:cluster{i32, i32, i32})  [unwired: 2 in]
            n473 = call "SeriellRead-11-15.vi"("SkalierungsfaktorHorst"=w734, "VorwortHorst"=w735, "error in"=w707, "Zwischenspeicher"=w736, "Senden?"=w729, "FPGA VI Reference In"=w717) -> ("Senden?"=w737:bool[], "Zwischenspeicher"=w710:string[], "error out"=w706:errorcluster)  [unwired: 3 in]
            "SeriellReadWrite" <- w706
          }
        }
      }
    }
    frame #2 {
      n474 = xnode "Read/Write Control"("FPGA VI Reference In"=w1264, "global stop"=TRUE) -> ("FPGA VI Reference Out"=w1263:refnum<k20>)  [unwired: 1 in, 1 out]
      n475 = xnode "Close FPGA VI Reference"("FPGA VI Reference In"=w1263) -> ()  [unwired: 1 in, 1 out]
    }
  }
